vi "DEFINE_HMI_v2.0.vi"() -> ()   [LabVIEW 2020]
uses:
  <vilib>/userdefined/High Color/IMAQdx.ctl
  Keyence CL-3000/Public/clusters/CL3IF_MEASUREMENT_DATA.ctl
  Keyence CL-3000/Public/clusters/CL3IF_OUTMEASUREMENT_DATA.ctl
  Keyence CL-3000/Public/enums/CL3IF_VALUE_INFO.ctl
  Keyence CL-3000/Public/enums/CL3IF_JUDGE_RESULT.ctl
  Supporting Files/Sensor Station States.ctl
  Keyence CL-3000/Public/clusters/CL3IF_ETHERNET_SETTING.ctl
  4961857f-4cb1-4452-8877-0132d1278599.vi
  8fbe439c-06e5-460e-a560-e938ce784f44.vi
  460a15f0-0b3a-4794-87ef-3f3f720a4f09.vi
  13309ec4-5ddb-4caa-9ccb-149c6c5ba2b7.vi
  <vilib>/WebDAVClient/Advanced/Get File.vi
  <vilib>/Utility/inputDevices.llb/keyboardAcquire.vi
  <vilib>/Utility/inputDevices.llb/closeKeyboard.vi
  Keyence CL-3000/Keyence CL-3000.lvlib
  <vilib>/vision/driver/NI_Vision_Acquisition_Software.lvlib
  <vilib>/WebDAVClient/NI_WebDAV.lvlib
panel:
  out "Encoder Value":ext
  in  "Display Tab":enum32{"SENSOR FEEDBACK"}(tab)
  out "Chromatic Confocal":dbl(graph)
  out "Laser Displacement (cRIO)":dbl(graph)
  out "Captured Image":T1(plugin-control)
  out "Camera Feed":T1(plugin-control)
  in  "Motion Tab":enum32{"POSITION", "MEASUREMENT"}(tab)
  in  "Run Program":bool
  in  "Select Program":string(combo)="NONE"
  out "1st Key":T2(ring)
  in  "Bottom Button":bool
  in  "Top Button":bool
  in  "Next Button":bool
  in  "Previous Button":bool
  in  "Up Button":bool
  in  "Down Button":bool
  in  "Jog Axes":bool
  in  "Menu Ring":string(combo)
  in  "Move":bool
  in  "Axis 2 Distance":dbl format="%.2g"
  in  "Axis 1 Distance":dbl format="%.2g"
  in  "Axis 0 Distance":dbl format="%.2g"
  in  "Axis 0 Speed":dbl format="%.2g"
  in  "Axis 1 Speed":dbl format="%.2g"
  in  "Axis 2 Speed":dbl format="%.2g"
  in  "Axis 1 Acc":dbl format="%.2g"
  in  "Axis 0 Acc":dbl format="%.2g"
  in  "Axis 2 Acc":dbl format="%.2g"
  in  "Set Parameters 2":bool
  in  "Axis 2 Jogspeed":dbl format="%.2g"
  in  "Axis 1 Jogspeed":dbl format="%.2g"
  in  "Axis 0 Jogspeed":dbl format="%.2g"
  in  "Capture Image":bool
  in  "Sensor":i32(ring) items=["Chromatic", "Laser"]
  in  "Chromatic Data \nLogging":bool
  out "Logged Data Points":u32
  out "Index End":u32
  out "Index Start":u32
  out "Suffix":string
  in  "Measurement\nAxis":i32(ring) items=["X Axis", "Y Axis"]
  in  "Travel Speed\n(mm/s)":dbl format="%.2g"
  in  "Set Parameters":bool
  in  "Track Offset\n(mm)":dbl format="%.2g"
  in  "Ramp Distance\n(mm)":dbl min=0.0 format="%.2g"
  in  "Num Tracks":i32
  in  "Evaluation Length\n(mm)":dbl max=40.0 format="%.2g"
  in  "Test Name":string
  in  "Laser Data\nLogging":bool
  out "Travel Dist":dbl
  in  "Travel Acc\n(mm/s2)":dbl format="%.2g"
  in  "Start Measurement":bool
  in  "STOP":bool
  in  "Setup Tab":enum32{"SETUP", "MONITORING", "ERRORS"}(tab)
  in  "Home Axes":bool
  in  "Enable Camera":bool
  in  "Enable Laser":bool
  in  "Camera Input":T3
  in  "Enable Chromatic":bool
  in  "IP Address":u8[](array[numeric])=[192, 168, 1, 1]
  in  "Port":u32
  in  "Timeout":u32=5000
  in  "Comm Interface":enum8{"USB", "ETHERNET"}(ring)
  in  "Device ID":i32 min=0 max=2
  out "IsOpen":bool
  in  "Connection?":refnum<k7>(container)
  in  "Connect  to Controller":bool=TRUE
  in  "Set Parameters":bool
  in  "Controller Connection Type":string(combo)="2"
  out "Controller Type":string
  out "Product Name":string
  out "Version":string
  out "Serial Port":fxp<+,3,3>
  in  "Axis Enable":bool
  in  "Save Directory":path
  out "Z Error":bool
  out "Y Error":bool
  out "X Error":bool
  out "Axis 2 Velocity":dbl format="%.3g"
  out "Axis 2 End Pos":dbl format="%.3g"
  out "Axis 2 Position":dbl format="%.3g"
  out "Axis 0 Position":dbl format="%.3f"
  out "Axis 0 End Pos":dbl format="%.3g"
  out "Axis 0 Velocity":dbl format="%.3g"
  out "Axis 1 Position":dbl format="%.3g"
  out "Axis 1 Velocity":dbl format="%.3g"
  out "Axis 1 End Pos":dbl format="%.3g"
  out "A0 Remaining":dbl format="%.3g"
  out "A1 Remaining":dbl format="%.3g"
  out "A2 Remaining":dbl format="%.3g"
  out "Loop Time (us)":u32
  out "Measurement Data":T4(array[cluster])=[{"Out No"=1, "Value"=0, "valueInfo"=enum."VALID", "judgeResult"=0}, {"Out No"=2, "Value"=0, "valueInfo"=enum."VALID", "judgeResult"=0}, {"Out No"=3, "Value"=0, "valueInfo"=enum."VALID", "judgeResult"=0}, {"Out No"=4, "Value"=0, "valueInfo"=enum."VALID", "judgeResult"=0}, {"Out No"=5, "Value"=0, "valueInfo"=enum."VALID", "judgeResult"=0}, {"Out No"=6, "Value"=0, "valueInfo"=enum."VALID", "judgeResult"=0}, {"Out No"=7, "Value"=0, "valueInfo"=enum."VALID", "judgeResult"=0}, {"Out No"=8, "Value"=0, "valueInfo"=enum."VALID", "judgeResult"=0}] {"judgeResult" items=["HI"=1, "GO"=2, "LO"=4, "**"=5, "--"=0]}
  out "Total Time Elapsed (s)":i32
  out "XY Graph":cluster{"X":dbl, "Y":dbl}[](graph)
  out "Controller  Error":errorcluster
  out "Z Axis Error":errorcluster
  out "Y Axis Error":errorcluster
  out "X Axis Error":errorcluster
  out "Chromatic Sensor Error":errorcluster
  out "Laser Sensor Error":errorcluster
  # "SET PARAMETERS"
  # "DIRECT MOTION"
  # "SPEED \n(mm/s)"
  # "ACC / DEC\n(mm/s2)"
  # "JOGSPEED \n(mm/s)"
  # "X AXIS"
  # "X AXIS"
  # "(mm)"
  # "Y AXIS"
  # "Y AXIS"
  # "(mm)"
  # "Z AXIS"
  # "Z AXIS"
  # "(mm)"
  # "AXIS JOGGING"
  # "XY AXES"
  # "Z AXIS"
  # "KEYBOARD"
  # "CONTROLLER PROGRAMS"
  # "Suffix will be auto-genereated for each measurement e.g. Test Name_01, Test Name_02, etc."
  # "MEASUREMENT PARAMETERS"
  # "CHROMATIC CONFOCAL"
  # "LASER DISPLACEMENT"
  # "CAMERA"
  # "CONTROLLER SETTINGS"
  # "CHROMATIC CONFOCAL SETTINGS"
  # "LASER DISPLACEMENT SETTINGS"
  # "CAMERA SETTINGS"
  # "AXIS FEEDBACK"
  # "Current Position \n(mm)"
  # "End Position \n(mm)"
  # "Travel Remaining \n(mm)"
  # "Velocity \n(mm/s2)"
  # "X AXIS"
  # "Y AXIS"
  # "Z AXIS"
  # "CONTROLLER"
  # "CHROMATIC CONFOCAL"
  # "CONTROLLER"
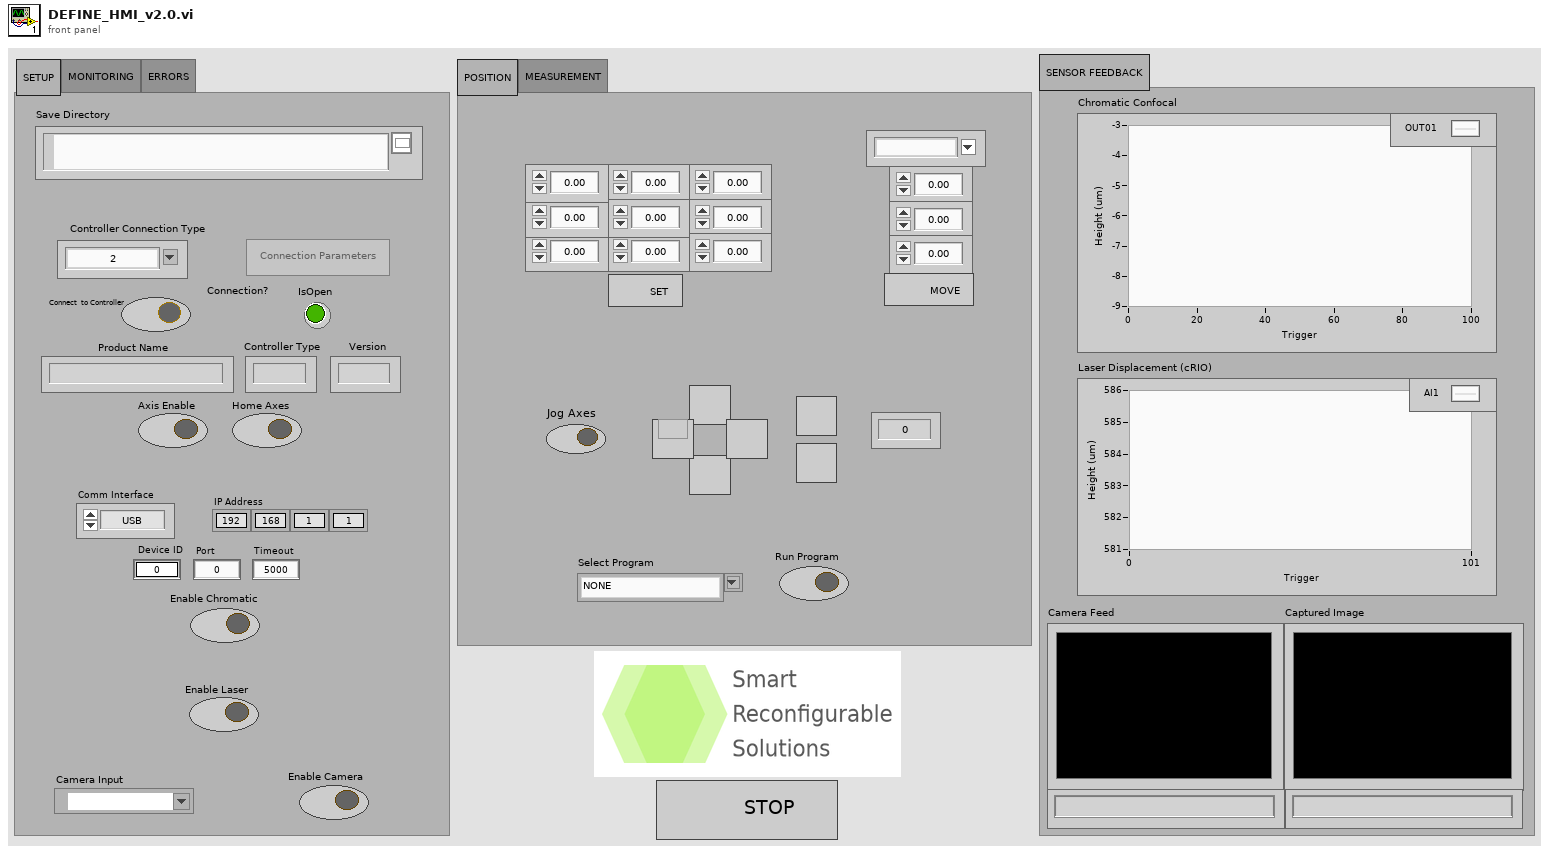
[diagram p1: front panel]
types:
  T1 = typedef "IMAQ Image.ctl" = refnum<image>
  T2 = enum16{"0", "1", "2", "3", "4", "5", "6", "7", "8", "9", "A", "B", "C", "D", "E", "F", "G", "H", "I", "J", "K", "L", "M", "N", "O", "P", "Q", "R", "S", "T", "U", "V", "W", "X", "Y", "Z", "F1", "F2", "F3", "F4", "F5", "F6", "F7", "F8", "F9", "F10", "F11", "F12", "F13", "F14", "F15", "ADD", "BACK", "BACKSLASH", "CAPITAL", "COMMA", "DECIMAL", "DELETE", "DIVIDE", "DOWN", "END", "EQUALS", "ESCAPE", "GRAVE (`)", "HOME", "INSERT", "LBRACKET", "LCONTROL", "LEFT", "L ALT", "LSHIFT", "LWIN", "MINUS", "MULTIPLY", "NEXT", "NUMLOCK", "NUMPAD_0", "NUMPAD_1", "NUMPAD_2", "NUMPAD_3", "NUMPAD_4", "NUMPAD_5", "NUMPAD_6", "NUMPAD_7", "NUMPAD_8", "NUMPAD_9", "PAUSE", "PERIOD", "PRIOR (PG UP)", "RBRACKET", "RCONTROL", "RETURN", "RIGHT", "R ALT", "RSHIFT", "RWIN", "SCROLL", "SEMICOLON", "SLASH", "SPACE", "SUBTRACT", "TAB", "UP", "ENTER (num pad)", "' (quote)"}
  T3 = typedef "IMAQdx.ctl" = refnum<k21>
  T4 = cluster{"Out No":i32, "Value":i32, "valueInfo":enum8{"VALID", "JUDGMENTSTANDBY", "INVALID", "OVERDISPRANGE_P", "OVERDISPRANGE_N"}, "judgeResult":u16}[]
  T5 = typedef "Sensor Station States.ctl" = enum16{"Initialise", "Acquire", "Visualise", "Log", "Save", "Check Time", "Idle", "Close"}
  T6 = enum16{"open", "replace", "create", "open or create", "replace or create", "replace or create with confirmation"}
  T7 = typedef "Keyence CL-3000.lvlib/CL3IF_ETHERNET_SETTING.ctl" = cluster{"IP Address":cluster{"IP1":u8, "IP2":u8, "IP3":u8, "IP4":u8}, "portNo":u32}
  T8 = typedef "Keyence CL-3000.lvlib/CL3IF_MEASUREMENT_DATA.ctl" = cluster{"addInfo":cluster{"triggerCount":u32, "pulseCount":i32}, "outMeasurementData":T9[]}
  T9 = typedef "Keyence CL-3000.lvlib/CL3IF_OUTMEASUREMENT_DATA.ctl" = cluster{"measurementValue":i32, "valueInfo":T10, "judgeResult":T11}
  T10 = typedef "Keyence CL-3000.lvlib/CL3IF_VALUE_INFO.ctl" = enum8{"VALID", "JUDGMENTSTANDBY", "INVALID", "OVERDISPRANGE_P", "OVERDISPRANGE_N"}
  T11 = typedef "Keyence CL-3000.lvlib/CL3IF_JUDGE_RESULT.ctl" = u8
  T12 = cluster{"IP Address":u8, "IP Address":u8, "IP Address":u8, "IP Address":u8}
  T13 = cluster{i32, "measurementValue":i32, "valueInfo":T10, "judgeResult":T11}
  T14 = typedef "NI_WebDAV.lvlib/SessionHandle.ctl" = refnum<k1>
  T15 = enum16{"0", "1", "2", "3", "4", "5", "6", "7", "8", "9", "A", "B", "C", "D", "E", "F", "G", "H", "I", "J", "K", "L", "M", "N", "O", "P", "Q", "R", "S", "T", "U", "V", "W", "X", "Y", "Z", "F1", "F2", "F3", "F4", "F5", "F6", "F7", "F8", "F9", "F10", "F11", "F12", "F13", "F14", "F15", "ADD", "BACK", "BACKSLASH", "CAPITAL", "COMMA", "DECIMAL", "DELETE", "DIVIDE", "DOWN", "END", "EQUALS", "ESCAPE", "GRAVE (`)", "HOME", "INSERT", "LBRACKET", "LCONTROL", "LEFT", "L ALT", "LSHIFT", "LWIN", "MINUS", "MULTIPLY", "NEXT", "NUMLOCK", "NUMPAD_0", "NUMPAD_1", "NUMPAD_2", "NUMPAD_3", "NUMPAD_4", "NUMPAD_5", "NUMPAD_6", "NUMPAD_7", "NUMPAD_8", "NUMPAD_9", "PAUSE", "PERIOD", "PRIOR (PG UP)", "RBRACKET", "RCONTROL", "RETURN", "RIGHT", "R ALT", "RSHIFT", "RWIN", "SCROLL", "SEMICOLON", "SLASH", "SPACE", "SUBTRACT", "TAB", "UP", "ENTER (num pad)", "' (quote)"}[]
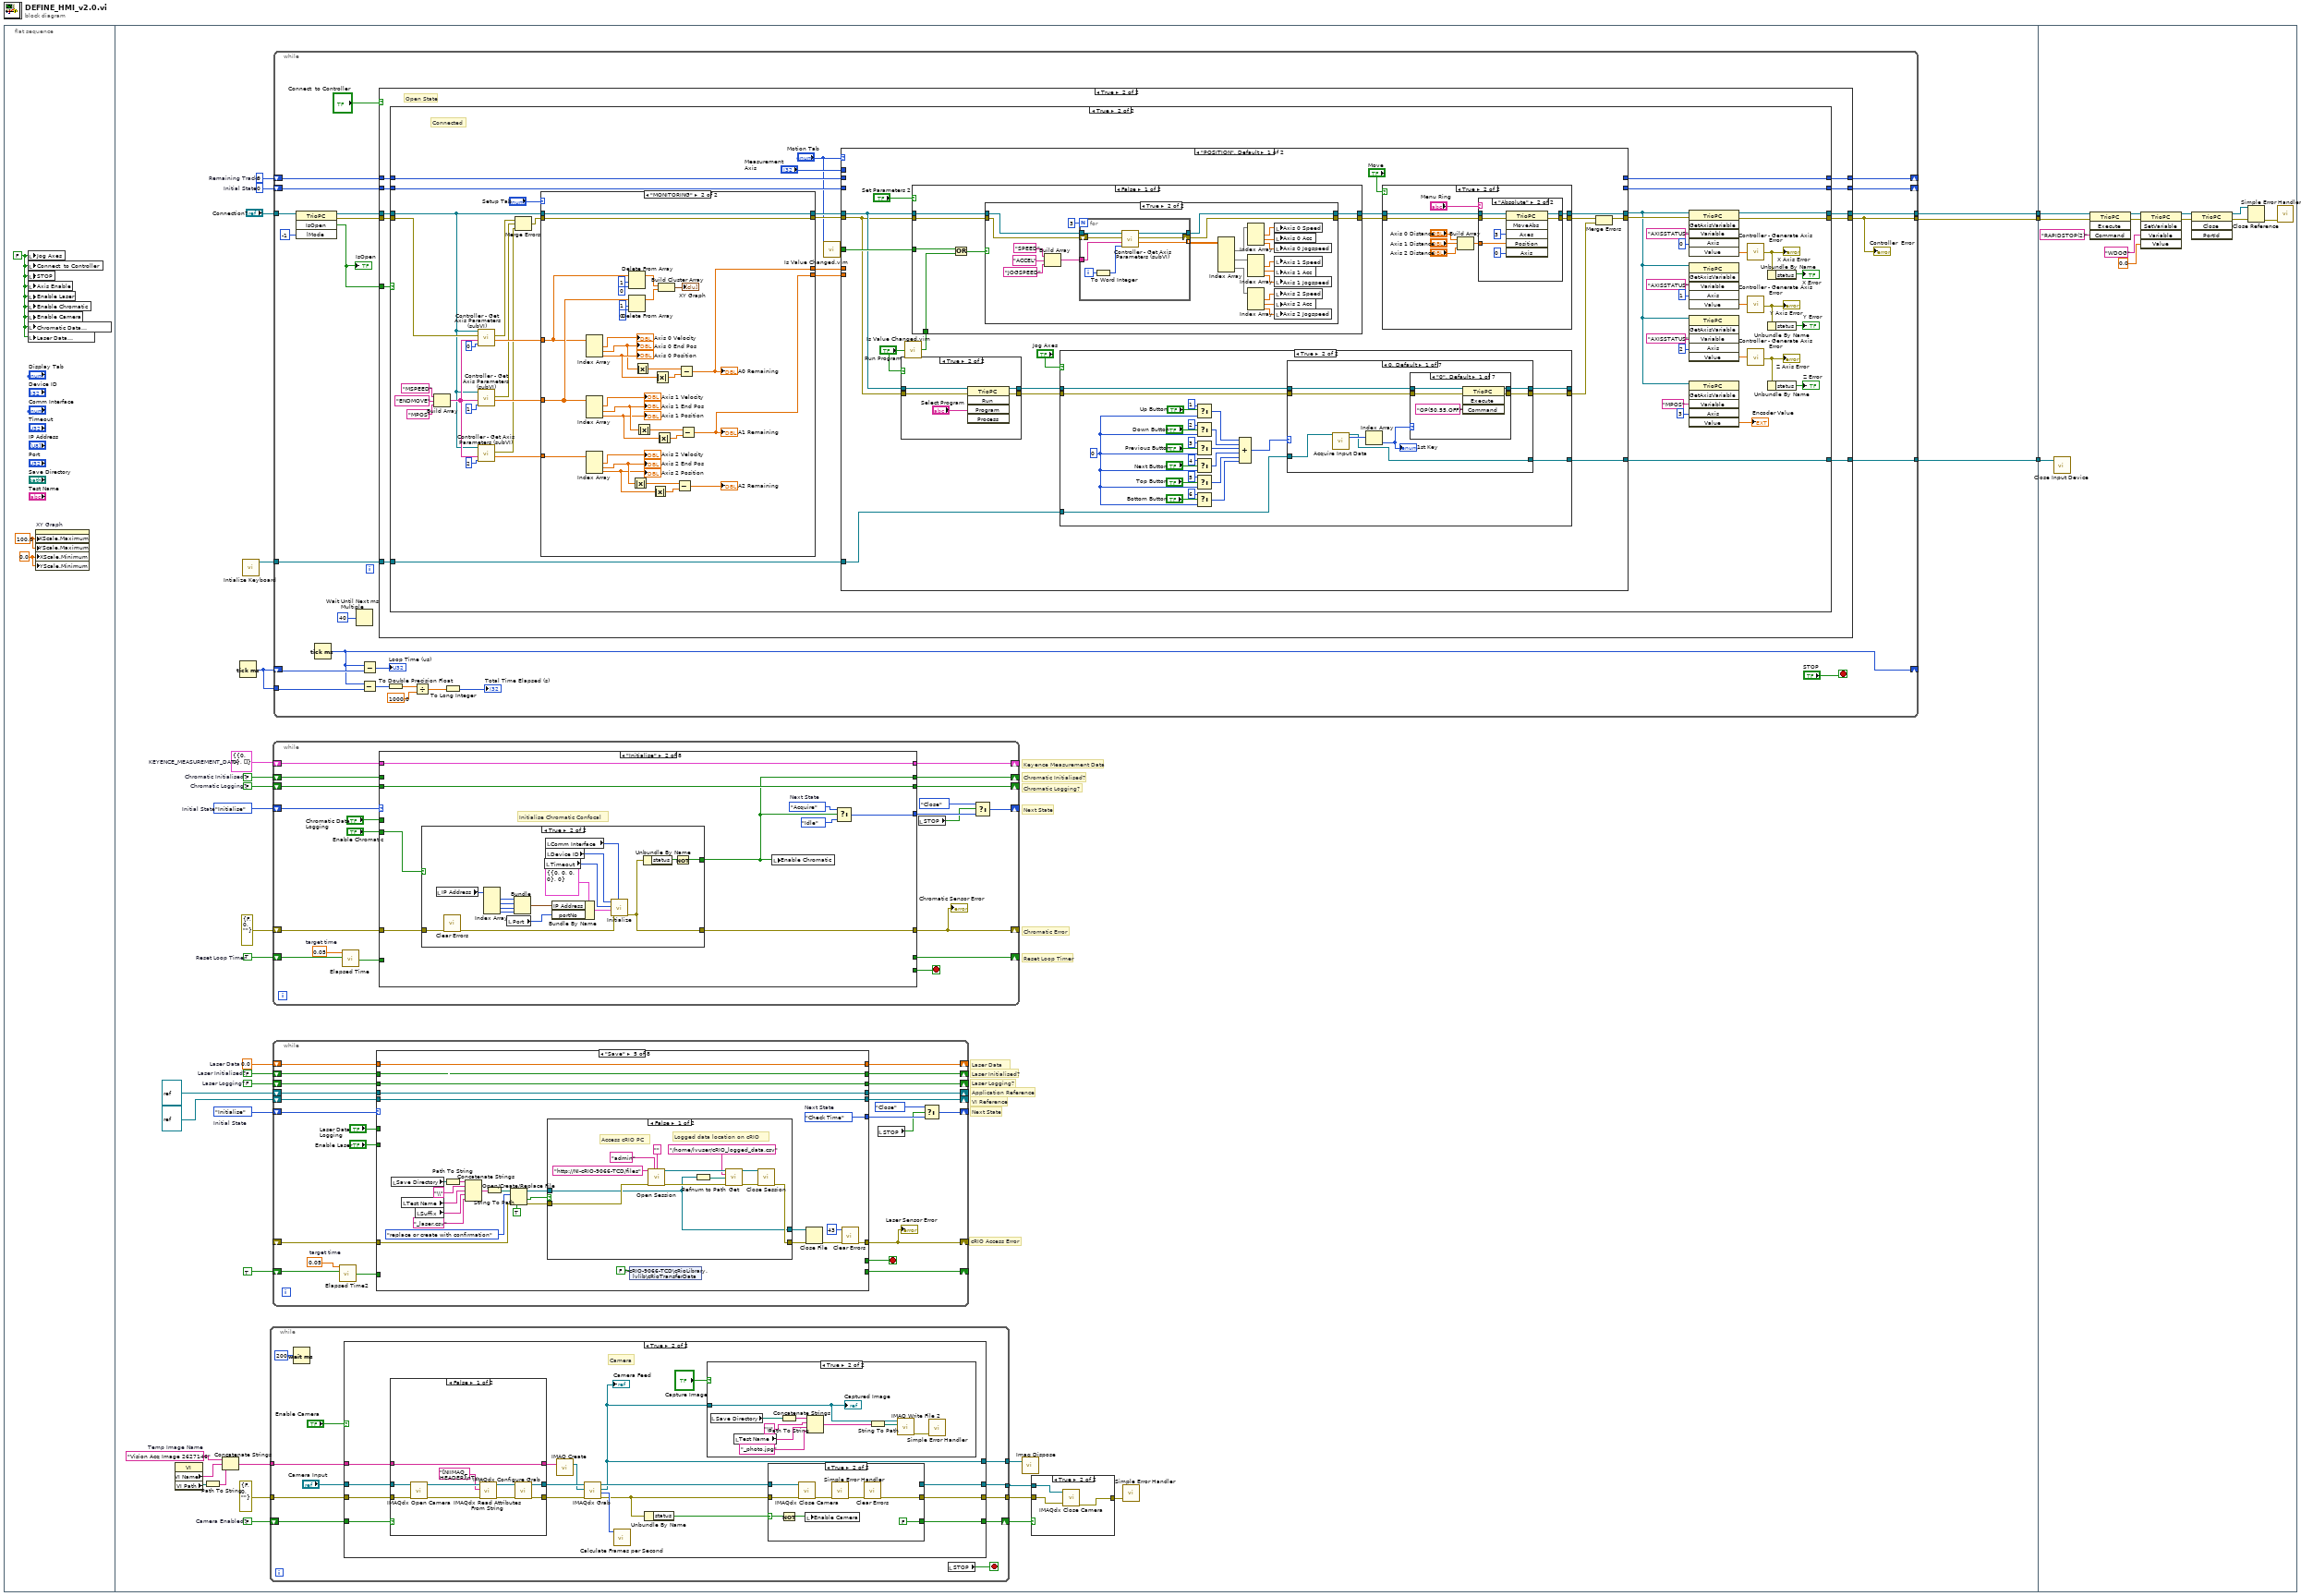
[diagram p0: block diagram]
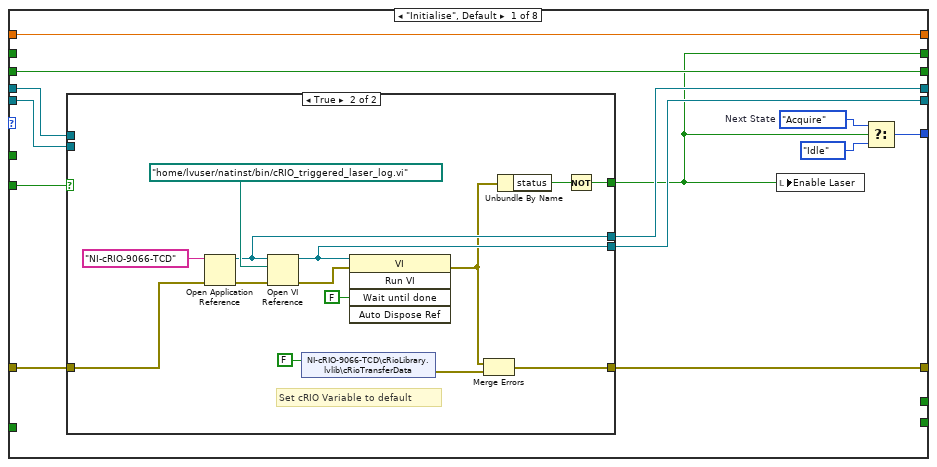
[diagram p2: hidden frame]
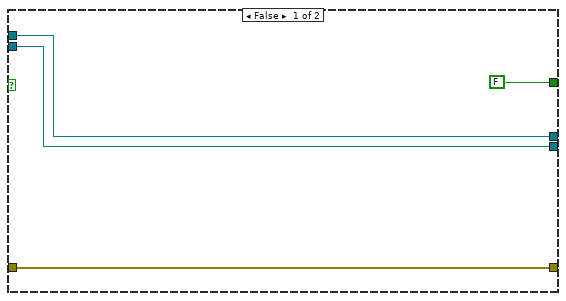
[diagram p3: hidden frame]
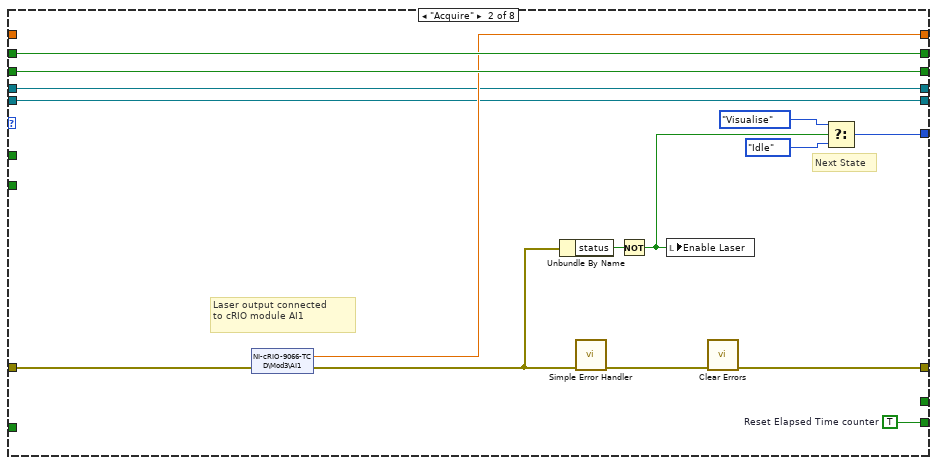
[diagram p4: hidden frame]
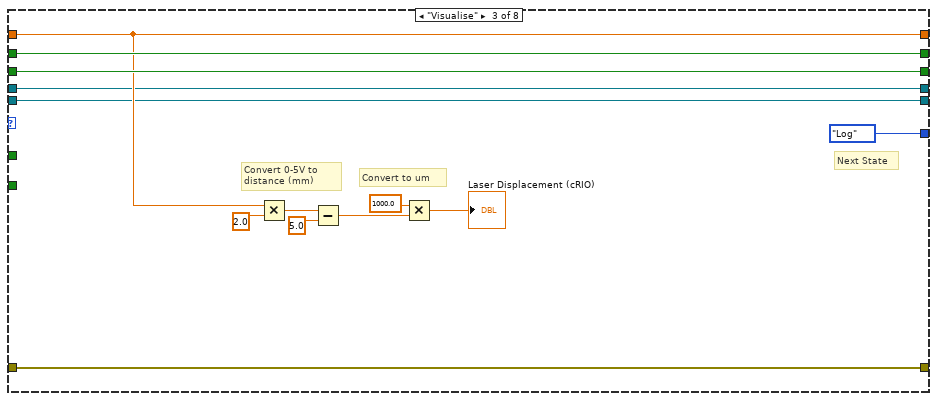
[diagram p5: hidden frame]
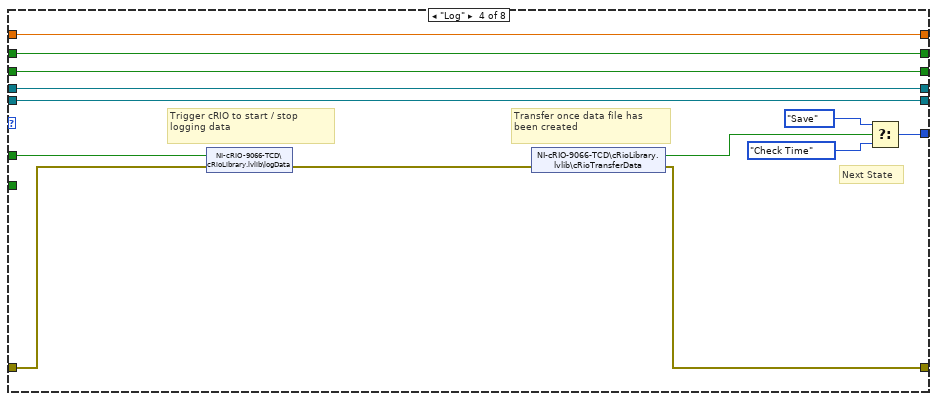
[diagram p6: hidden frame]
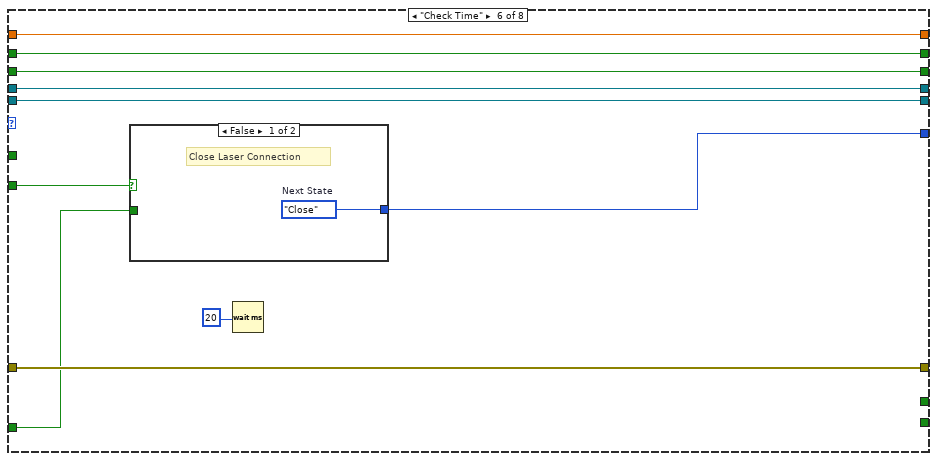
[diagram p8: hidden frame]
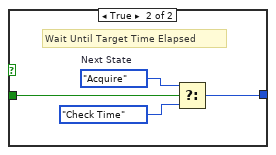
[diagram p9: hidden frame]
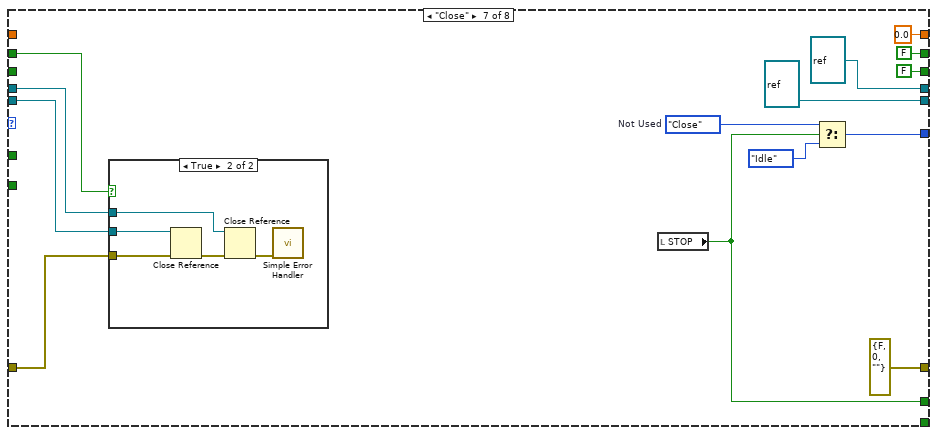
[diagram p10: hidden frame]
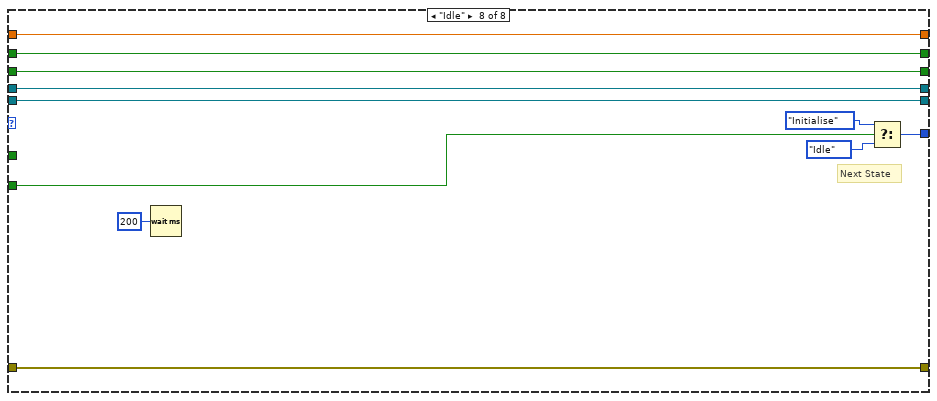
[diagram p12: hidden frame]
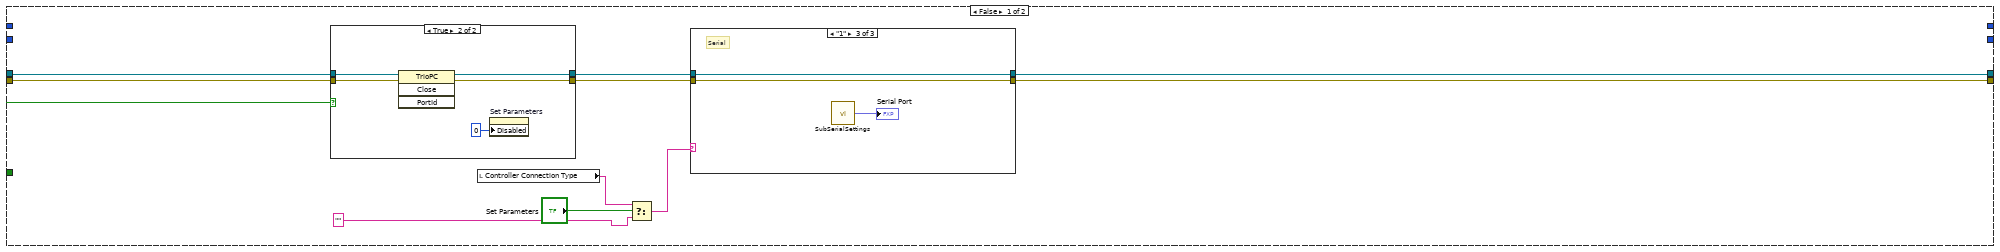
[diagram p13: hidden frame]
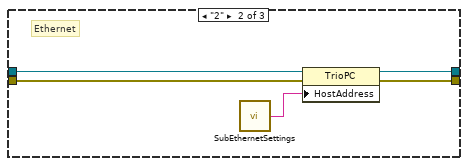
[diagram p16: hidden frame]
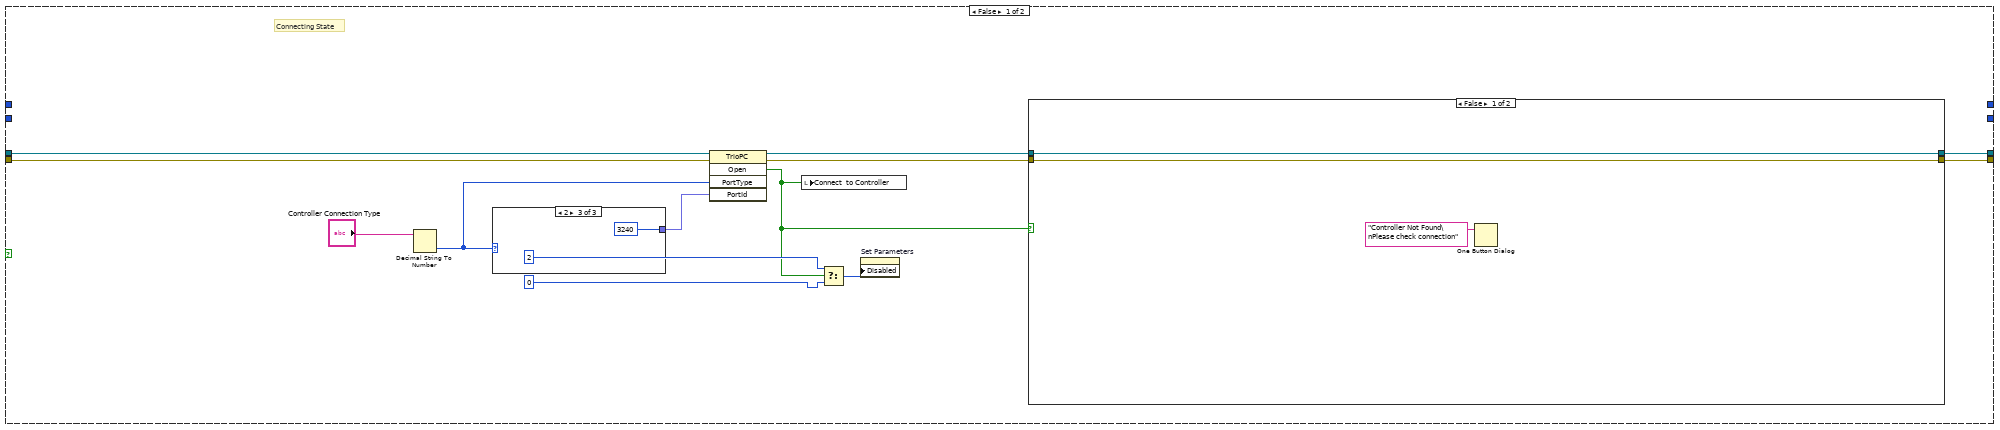
[diagram p17: hidden frame]
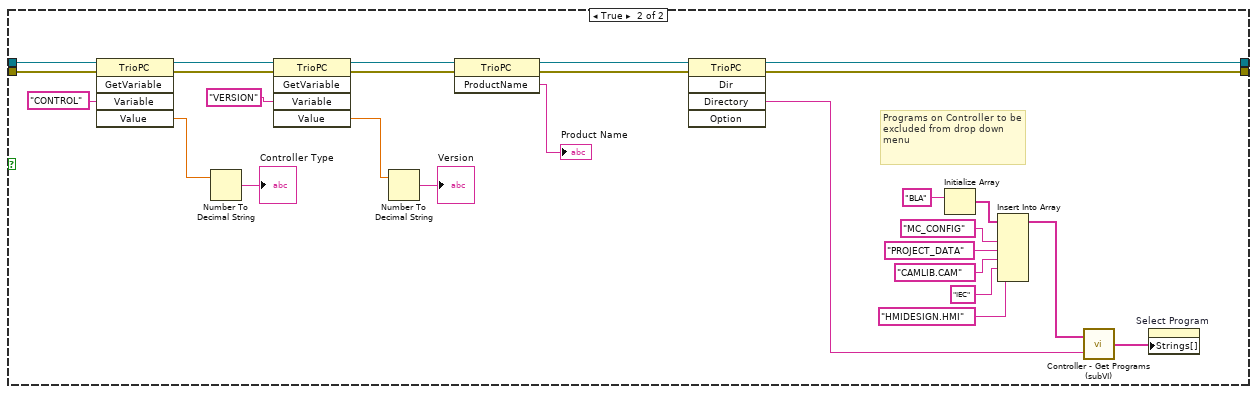
[diagram p18: hidden frame]
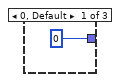
[diagram p19: hidden frame]
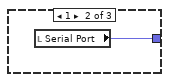
[diagram p20: hidden frame]
diagram:
  n1 = flat-sequence {
    tunnel: [w38] -> w3
    tunnel: [w37] -> w2
    tunnel: [w34] -> w1
    tunnel: w3 -> [w1152]
    tunnel: w2 -> [w1153]
    tunnel: w1 -> [w1154]
    frame #0 {
      w6 = 0.0 ("X Scale.Range:Minimum")
      w5 = 100.0 ("X Scale.Range:Maximum")
      w4 = FALSE ("Jog Axes")
      n2 = local write "Jog Axes"(w4) -> ()
      n3 = local write "Connect  to Controller"(w4) -> ()
      n4 = local write "STOP"(w4) -> ()
      n5 = local write "Axis Enable"(w4) -> ()
      n6 = local write "Enable Laser"(w4) -> ()
      n7 = local write "Enable Chromatic"(w4) -> ()
      n8 = local write "Enable Camera"(w4) -> ()
      n9 = local write "Chromatic Data \nLogging"(w4) -> ()
      n10 = local write "Laser Data\nLogging"(w4) -> ()
      n11 = property on="XY Graph" class="XYGraph (strict)"("XScale.Maximum"=w5, "YScale.Maximum"=w5, "XScale.Minimum"=w6, "YScale.Minimum"=w6) -> ()  [unwired: 2 in, 2 out]
    }
    frame #1 {
      w9 = 0.0  # Laser Data
      w10 = FALSE  # Laser Initialised?
      w13 = FALSE  # Laser Logging?
      w11 = Sensor_Station_States."Initialise"  # Initial State
      w14 = 0  # Remaining Tracks
      w15 = 0  # Initial State
      w18 = "Vision Acq Image 2627146"  # Temp Image Name
      w17 = FALSE  # Camera Enabled?
      w28 = FALSE  # Chromatic Initialised?
      w30 = FALSE  # Chromatic Logging?
      w31 = TRUE  # Reset Loop Timer
      w32 = T8 {"addInfo"={"triggerCount"=0, "pulseCount"=0}, "outMeasurementData"=[]}  # KEYENCE_MEASUREMENT_DATA
      w33 = Sensor_Station_States."Initialise"  # Initial State
      # "VI Reference"
      # "Application Reference"
      # "cRIO Access Error"
      # "Next State"
      # "Laser Logging?"
      # "Laser Initialised?"
      # "Laser Data"
      # "Reset Loop Timer"
      # "Chromatic Error"
      # "Next State"
      # "Keyence Measurement Data"
      # "Chromatic Logging?"
      # "Chromatic Initialised?"
      n12 = property class="VI"() -> ("VI Name"=w21:string, "VI Path"=w22:path)  [unwired: 2 in, 2 out]
      n13 = Path To String(path=w22) -> (string=w20:string)
      n14 = Concatenate Strings(w18, w21, w20) -> (w23:string)
      n15 = Tick Count (ms)() -> (millisecond timer value=w36:u32)
      n16 = call <vilib>:"Intialize Keyboard.vi"() -> ("device ID"=w35:refnum<k1>)  [unwired: 1 in, 10 out]
      n17 = while {
        tunnel: [w901] -> w19
        tunnel: [w900] -> w25
        shift-right: [w892] -> w27
        shift-left: w17 -> [w896]
        tunnel: errorcluster {"status"=FALSE, "code"=0, "source"=""} ("error in") -> [w894]
        tunnel: w23 -> [w895]
        tunnel: [w891] -> w24
        stop <- w897 stop-if-true
        n18 = Wait (ms)(milliseconds to wait=u32 200) -> ()  [unwired: 1 out]
        n19 = case shown="True" "Enable Camera" {
          tunnel: [w903 w920] -> w900
          tunnel: [_ w914] -> w901
          tunnel: w896 -> [w902 w913]
          tunnel: w895 -> [_ w909]
          tunnel: w894 -> [w903 w912]
          tunnel: "Camera Input" -> [w904 w908]
          tunnel: [w902 w906] -> w892
          tunnel: [w904 w905] -> w891
          frame False {
          }
          frame True {
            # "Camera"
            n20 = case shown="False" w913 {
              tunnel: [w931 w933] -> w916
              tunnel: [w930 w932] -> w915
              tunnel: w912 -> [w925 w932]
              tunnel: [w924 w934] -> w910
              tunnel: w909 -> [w924 w934]
              tunnel: w908 -> [w923 w933]
              frame False {
                n21 = call <vilib>:"IMAQdx Open Camera.vi"("error in"=w925, "Session In"=w923) -> ("error out"=w928:errorcluster, "Session Out"=w929:T3)  [unwired: 1 in, 7 out]
                n22 = call <vilib>:"IMAQdx Read Attributes From String.vi"("error in"=w928, "Attributes String In"="[NIIMAQ_HEADER]\nType = 2\nVersion = 8\n\n[CAMERA_DATA]\nAcquisitionAttributes::Bayer::Algorithm = \"Bilinear\"\nAcquisitionAttributes::Bayer::GainB = \"1\"\nAcquisitionAttributes::Bayer::GainG = \"1\"\nAcquisitionAttributes::Bayer::GainR = \"1\"\nAcquisitionAttributes::Bayer::Pattern = \"Use hardware value\"\nAcquisitionAttributes::BitsPerPixel = \"Use hardware value\"\nAcquisitionAttributes::HardwareMaximumQueuedBufferCount = \"1000\"\nAcquisitionAttributes::HardwareRequeueBufferListThreshold = \"50\"\nAcquisitionAttributes::IgnoreFirstFrame = \"false\"\nAcquisitionAttributes::ImageDecoderCopyMode = \"Auto\"\nAcquisitionAttributes::OutputImageType = \"Auto\"\nAcquisitionAttributes::OverwriteMode = \"Get Newest\"\nAcquisitionAttributes::PixelSignedness = \"Use hardware value\"\nAcquisitionAttributes::ReceiveTimestampMode = \"None\"\nAcquisitionAttributes::ShiftPixelBits = \"false\"\nAcquisitionAttributes::SwapPixelBytes = \"false\"\nAcquisitionAttributes::Timeout = \"5000\"\nAcquisitionAttributes::VerticalMirror = \"false\"\nAcquisitionAttributes::VideoMode = \"640x480 YUY2 30.00fps\"\nCameraAttributes::BacklightCompensation::Mode = \"Manual\"\nCameraAttributes::BacklightCompensation::Value = \"true\"\nCameraAttributes::Brightness::Mode = \"Manual\"\nCameraAttributes::Brightness::Value = \"0\"\nCameraAttributes::Contrast::Mode = \"Manual\"\nCameraAttributes::Contrast::Value = \"0.179999999999999993\"\nCameraAttributes::Exposure::Mode = \"Auto\"\nCameraAttributes::Gain::Mode = \"Manual\"\nCameraAttributes::Gain::Value = \"1\"\nCameraAttributes::Gamma::Mode = \"Manual\"\nCameraAttributes::Gamma::Value = \"1.5\"\nCameraAttributes::Hue::Mode = \"Manual\"\nCameraAttributes::Hue::Value = \"0\"\nCameraAttributes::Saturation::Mode = \"Manual\"\nCameraAttributes::Saturation::Value = \"8\"\nCameraAttributes::Sharpness::Mode = \"Manual\"\nCameraAttributes::Sharpness::Value = \"3\"\nCameraAttributes::WhiteBalance::Mode = \"Auto\"\n" ("Attributes"), "Session In"=w929) -> ("error out"=w926:errorcluster, "Session Out"=w927:T3)  [unwired: 7 out]
                n23 = call <vilib>:"IMAQdx Configure Grab.vi"("error in"=w926, "Session In"=w927) -> ("error out"=w930:errorcluster, "Session Out"=w931:T3)  [unwired: 1 in, 7 out]
              }
              frame True {
                # "Camera Initialised"
              }
            }
            n24 = call "IMAQ Create"("Image Name"=w910) -> ("New Image"=w911:T1)  [unwired: 3 in, 2 out]
            n25 = call <vilib>:"IMAQdx Grab.vi"("error in"=w915, "Image In"=w911, "Session In"=w916) -> ("error out"=w917:errorcluster, "Buffer Number Out"=w918:u32, "Image Out"=w914:T1, "Session Out"=w919:T3)  [unwired: 1 in, 4 out]
            "Camera Feed" <- w914
            n26 = call <vilib>:"Calculate Frames per Second.vi"("Buffer Number"=w918) -> ()  [unwired: 2 in, 9 out]
            n27 = Unbundle By Name(w917) -> ("status"=w907:bool)
            n28 = case shown="True" "Capture Image" {
              tunnel: w914 -> [_ w954]
              frame False {
              }
              frame True {
                n29 = local read "Save Directory"() -> (w950:path)
                n30 = local read "Test Name"() -> (w952:string)
                n31 = Path To String(path=w950) -> (string=w951:string)
                n32 = Concatenate Strings(w951, "\\" ("string"), w952, "_photo.jpg" ("string")) -> (w949:string)
                n33 = String To Path(string=w949) -> (path=w946:path)
                n34 = call-poly "IMAQ Write File 2"("File Path"=w946, "Image"=w954) -> ("error out"=w953:errorcluster)  [unwired: 8 in, 1 out]
                n35 = call <vilib>:"Simple Error Handler.vi"("error in (no error)"=w953) -> ()  [unwired: 4 in, 5 out]
                "Captured Image" <- w954
              }
            }
            n36 = case "Case Structure_template1" shown="True" w907 {
              selector: w907 -> [_ w940]
              tunnel: [w937 w941] -> w920
              tunnel: w917 -> [w937 w945]
              tunnel: w919 -> [w935 w943]
              tunnel: [TRUE FALSE] -> w906
              tunnel: [w935 _] -> w905
              frame False {
              }
              frame True {
                n37 = Not(x=w940) -> (.not. x?=w939:bool)
                n38 = call <vilib>:"IMAQdx Close Camera.vi"("error in"=w945, "Session In"=w943) -> ("error out"=w944:errorcluster)  [unwired: 9 out]
                n39 = local write "Enable Camera"(w939) -> ()
                n40 = call <vilib>:"Simple Error Handler.vi"("error in (no error)"=w944) -> ("error out"=w942:errorcluster)  [unwired: 4 in, 4 out]
                n41 = call <vilib>:"Clear Errors.vi"("error in (no error)"=w942) -> ("error out"=w941:errorcluster)  [unwired: 5 in, 1 out]
              }
            }
          }
        }
        n42 = local read "STOP"() -> (w897:bool)
      }
      n43 = while {
        shift-right: [w960] -> _
        shift-left: w33 -> [w974]
        shift-right: [w972] -> _
        shift-left: w32 -> [w973]
        shift-right: [w968] -> _
        shift-left: w31 -> [w970]
        shift-right: [w966] -> _
        shift-left: w30 -> [w967]
        shift-right: [w955] -> _
        shift-left: errorcluster {"status"=FALSE, "code"=0, "source"=""} ("error constant") -> [w965]
        shift-right: [w964] -> _
        shift-left: w28 -> [w963]
        stop <- w959 stop-if-true
        w971 = 0.05  # target time
        n44 = call "Elapsed Time"("Time Target (s)"=w971, "Reset"=w970) -> ("Time has Elapsed"=w969:bool)  [unwired: 10 in, 7 out]
        n45 = case shown="\"Initialise\"" w974 {
          tunnel: w973 -> [w982 w992 _ w1028 w1047 w1095 w1120 _]
          tunnel: w965 -> [w976 w988 w1017 w1031 w1050 w1081 w1123 w1141]
          tunnel: [w982 w992 w1013 w1028 w1047 w1095 w1120 T8 {"addInfo"={"triggerCount"=0, "pulseCount"=0}, "outMeasurementData"=[]} ("KEYENCE_MEASUREMENT_DATA")] -> w972
          tunnel: [w979 w990 w1016 Sensor_Station_States."Log" ("Next State") w1043 w1086 w1121 w1135] -> w962
          tunnel: w969 -> [_ _ _ _ _ _ w1122 _]
          tunnel: [_ _ w1019 _ _ _ _ _] -> w968
          tunnel: w967 -> [w975 w989 w1018 w1030 w1051 w1084 w1125 _]
          tunnel: [w975 w989 w1018 w1030 w1049 w1084 w1125 FALSE ("Chromatic Logging?")] -> w966
          tunnel: [w976 w984 w1014 w1031 w1040 w1082 w1123 errorcluster {"status"=FALSE, "code"=0, "source"=""} ("error constant")] -> w955
          tunnel: [w983 w985 w1012 w1032 w1048 w1085 w1124 FALSE] -> w964
          tunnel: w963 -> [w983 _ w1012 w1032 w1048 w1085 w1124 w1134]
          tunnel: [_ _ _ _ _ _ _ w1132] -> w959
          tunnel: "Enable Chromatic" -> [w978 w986 _ _ _ _ w1119 _]
          tunnel: "Chromatic Data \nLogging" -> [_ _ _ _ w1042 _ _ _]
          frame "Idle", Default {
            w981 = Sensor_Station_States."Initialise"  # Next State
            n46 = Wait (ms)(milliseconds to wait=u32 200) -> ()  [unwired: 1 out]
            n47 = Select(t=w981, s=w978, f=Sensor_Station_States."Idle" ("Next State")) -> (s? t:f=w979:T5)
          }
          frame "Initialise" {
            w991 = Sensor_Station_States."Acquire"  # Next State
            # "Initialise Chromatic Confocal"
            n48 = case shown="True" w986 {
              tunnel: [w993 w998] -> w984
              tunnel: [FALSE w997] -> w985
              tunnel: w988 -> [w993 w999]
              frame False {
              }
              frame True {
                n49 = local read "IP Address"() -> (w1001:u8[])
                n50 = call <vilib>:"Clear Errors.vi"("error in (no error)"=w999) -> ("error out"=w995:errorcluster)  [unwired: 5 in, 1 out]
                n51 = Index Array(array=w1001) -> (element #1=w1006:u8, element #2=w1007:u8, element #3=w1008:u8, element #4=w1009:u8)  [unwired: 4 in]
                n52 = local read "Port"() -> (w1000:u32)
                n53 = Bundle("IP Address"=w1006, "IP Address"=w1007, "IP Address"=w1008, "IP Address"=w1009) -> (w1010:T12)  [unwired: 1 in]
                n54 = local read "Timeout"() -> (w1002:u32)
                n55 = local read "Comm Interface"() -> (w1003:enum8{"USB", "ETHERNET"})
                n56 = local read "Device ID"() -> (w1004:i32)
                n57 = Bundle By Name(cluster=T7 {"IP Address"={"IP1"=0, "IP2"=0, "IP3"=0, "IP4"=0}, "portNo"=0} ("ethernetSetting"), "IP Address"=w1010, "portNo"=w1000) -> (w1011:T7)
                n58 = call "Initialize.vi"("Comm Interface"=w1003, "error in (no error)"=w995, "ethernetSetting"=w1011, "timeout"=w1002, "deviceId"=w1004) -> ("error out"=w998:errorcluster)  [unwired: 6 in]
                n59 = Unbundle By Name(w998) -> ("status"=w996:bool)
                n60 = Not(x=w996) -> (.not. x?=w997:bool)
              }
            }
            n61 = local write "Enable Chromatic"(w985) -> ()
            n62 = Select(t=w991, s=w985, f=Sensor_Station_States."Idle" ("Next State")) -> (s? t:f=w990:T5)
          }
          frame "Acquire" {
            w1016 = Sensor_Station_States."Visualise"  # Next State
            w1019 = TRUE  # Reset Elapsed Time counter
            n63 = local read "Device ID"() -> (w1015:i32)
            n64 = call "CL3IF_GetMeasurementData.vi"("error in"=w1017, "deviceId"=w1015) -> ("error out"=w1014:errorcluster, "MEASUREMENT_DATA"=w1013:T8)  [unwired: 8 in]
          }
          frame "Visualise" {
            n65 = Unbundle By Name(w1028) -> ("outMeasurementData"=w1026:T9[])
            n66 = Index Array(array=w1026, index=0) -> (element=w1025:T9)
            n67 = for {
              tunnel: w1026 -> [w1039] mode=indexing
              tunnel: [w1038] -> w1027 mode=indexing
              i -> [w1037]
              n68 = Unbundle By Name(w1039) -> ("measurementValue"=w1033:i32, "valueInfo"=w1035:T10, "judgeResult"=w1034:T11)
              n69 = Increment(x=w1037) -> (x+1=w1036:i32)
              n70 = Bundle(w1036, "measurementValue"=w1033, "valueInfo"=w1035, "judgeResult"=w1034) -> (w1038:T13)  [unwired: 1 in]
            }
            "Measurement Data" <- w1027
            n71 = Unbundle By Name(w1025) -> ("measurementValue"=w1024:i32)
            n72 = To Double Precision Float(number=w1024) -> (double precision float=w1020:dbl)
            n73 = Divide(x=w1020, y=1000.0) -> (x/y=→"Chromatic Confocal":dbl)
          }
          frame "Log" {
            w1045 = Sensor_Station_States."Save"  # Next State
            n74 = local read "Device ID"() -> (w1041:i32)
            n75 = case shown="False" w1042 {
              tunnel: w1051 -> [w1056 w1070]
              tunnel: w1050 -> [w1057 w1069]
              tunnel: [w1055 w1068] -> w1040
              tunnel: [FALSE TRUE] -> w1049
              tunnel: [w1053 FALSE ("conSaveData")] -> w1046
              tunnel: w1041 -> [w1052 w1065]
              frame False {
                n76 = case shown="True" w1056 {
                  tunnel: w1057 -> [w1059 w1063]
                  tunnel: [w1059 w1061] -> w1055
                  tunnel: [FALSE ("conSaveData") TRUE ("conSaveData")] -> w1053
                  tunnel: w1052 -> [_ w1060]
                  frame False {
                    # "Not Logging\nDo nothing"
                  }
                  frame True {
                    # "Move to Save State"
                    # "Stop Logging & Record Data Index"
                    n77 = call "CL3IF_GetTrendIndex.vi"("error in"=w1063, "deviceId"=w1060) -> ("error out"=w1061:errorcluster, "index"=→"Index End":u32)  [unwired: 8 in]
                  }
                }
              }
              frame True {
                n78 = case shown="False" w1070 {
                  tunnel: w1069 -> [w1073 w1075]
                  tunnel: [w1072 w1075] -> w1068
                  tunnel: w1065 -> [w1071 _]
                  frame False {
                    # "Start Logging"
                    n79 = call "CL3IF_GetTrendIndex.vi"("error in"=w1073, "deviceId"=w1071) -> ("error out"=w1072:errorcluster, "index"=→"Index Start":u32)  [unwired: 8 in]
                  }
                  frame True {
                    # "Currently Logging\nDo nothing"
                  }
                }
              }
            }
            n80 = Select(t=w1045, s=w1046, f=Sensor_Station_States."Check Time" ("Next State")) -> (s? t:f=w1043:T5)
          }
          frame "Save" {
            w1086 = Sensor_Station_States."Check Time"  # Next State
            n81 = local read "Save Directory"() -> (w1092:path)
            n82 = local read "Index Start"() -> (w1094:u32)
            n83 = local read "Index End"() -> (w1093:u32)
            n84 = local read "Test Name"() -> (w1089:string)
            n85 = local read "Suffix"() -> (w1076:string)
            n86 = local read "Device ID"() -> (w1083:i32)
            n87 = Path To String(path=w1092) -> (string=w1091:string)
            n88 = Concatenate Strings(w1091, "\\" ("string"), w1089, w1076, "_confocal.csv" ("string")) -> (w1088:string)
            n89 = Subtract(x=w1093, y=w1094) -> (x-y=w1102:u32)
            "Logged Data Points" <- w1102
            n90 = String To Path(string=w1088) -> (path=w1087:path)
            n91 = call "CL3IF_GetTrendData.vi"("requestDataCount"=w1102, "index"=w1094, "deviceId"=w1083) -> ("measurementData"=w1101:T8[])  [unwired: 4 in, 4 out]
            n92 = Open/Create/Replace File(file path (use dialog)=w1087, operation (0:open)=T6."replace or create with confirmation") -> (refnum out=w1100:refnum<file>, error out=w1097:errorcluster)  [unwired: 4 in, 1 out]
            n93 = for {
              tunnel: w1101 -> [w1118] mode=indexing
              tunnel: w1100 -> [w1107]
              tunnel: [w1105] -> w1099
              tunnel: w1097 -> [w1104]
              tunnel: [w1103] -> w1096
              n94 = Unbundle By Name(w1118) -> ("outMeasurementData"=w1116:T9[])
              n95 = Index Array(array=w1116, index=0) -> (element=w1115:T9)
              n96 = Unbundle By Name(w1115) -> ("measurementValue"=w1112:i32)
              n97 = To Double Precision Float(number=w1112) -> (double precision float=w1113:dbl)
              n98 = Divide(x=w1113, y=1000.0) -> (x/y=w1111:dbl)
              n99 = Format Into String(format string="%.6f%s", error in=w1104, w1111, "\r\n") -> (resulting string=w1108:string, error out=w1106:errorcluster)  [unwired: 1 in]
              n100 = Write to Text File(file (use dialog)=w1107, text=w1108, error in=w1106) -> (refnum out=w1105:refnum<file>, error out=w1103:errorcluster)  [unwired: 1 in, 1 out]
            }
            n101 = Close File(refnum=w1099, error in=w1096) -> (error out=w1079:errorcluster)  [unwired: 1 out]
            n102 = call <vilib>:"Clear Errors.vi"("error in (no error)"=w1079, "specific error code to clear (0: all)"=43) -> ("error out"=w1078:errorcluster)  [unwired: 4 in, 1 out]
            n103 = Merge Errors(w1078, w1081) -> (w1082:errorcluster)
          }
          frame "Check Time" {
            n104 = case shown="True" w1119 {
              tunnel: w1122 -> [_ w1129]
              tunnel: [w1127 w1128] -> w1121
              frame False {
                w1127 = Sensor_Station_States."Close"  # Next State
                # "Close Chromatic Connection"
              }
              frame True {
                w1130 = Sensor_Station_States."Acquire"  # Next State
                # "Wait Until Target Time Elapsed"
                n105 = Select(t=w1130, s=w1129, f=Sensor_Station_States."Check Time" ("Next State")) -> (s? t:f=w1128:T5)
              }
            }
            n106 = Wait (ms)(milliseconds to wait=u32 10) -> ()  [unwired: 1 out]
          }
          frame "Close" {
            w1137 = Sensor_Station_States."Close"  # Not Used
            n107 = case shown="True" w1134 {
              tunnel: w1141 -> [_ w1143]
              frame False {
              }
              frame True {
                n108 = local read "Device ID"() -> (w1142:i32)
                n109 = call "Close.vi"("error in (no error)"=w1143, "deviceId"=w1142) -> ()  [unwired: 9 in, 1 out]
              }
            }
            n110 = local read "STOP"() -> (w1132:bool)
            n111 = Select(t=w1137, s=w1132, f=Sensor_Station_States."Idle" ("Next State")) -> (s? t:f=w1135:T5)
          }
        }
        "Chromatic Sensor Error" <- w955
        n112 = local read "STOP"() -> (w956:bool)
        n113 = Select(t=Sensor_Station_States."Close" ("Next State"), s=w956, f=w962) -> (s? t:f=w960:T5)
      }
      n114 = while {
        shift-right: [w51] -> _
        shift-left: w11 -> [w63]
        shift-right: [w59] -> _
        shift-left: TRUE -> [w61]
        shift-right: [w57] -> _
        shift-left: w13 -> [w58]
        shift-right: [w44] -> _
        shift-left: _ -> [w56]
        shift-right: [w55] -> _
        shift-left: w10 -> [w54]
        shift-right: [w47] -> _
        shift-left: w9 -> [w46]
        shift-right: [w42] -> _
        shift-left: refnum<vi> refnum ("application reference") -> [w41]
        shift-right: [w43] -> _
        shift-left: refnum<vi> refnum -> [w40]
        stop <- w50 stop-if-true
        w62 = 0.05  # target time
        n115 = call "Elapsed Time2"("Time Target (s)"=w62, "Reset"=w61) -> ("Time has Elapsed"=w60:bool)  [unwired: 10 in, 7 out]
        n116 = case shown="\"Save\"" w63 {
          tunnel: w56 -> [w70 w108 w121 w127 w140 w182 w194 w215]
          tunnel: [w75 w98 Sensor_Station_States."Log" ("Next State") w133 w161 w179 w199 w217] -> w53
          tunnel: w60 -> [_ _ _ _ _ w180 _ _]
          tunnel: [_ w109 _ _ _ _ _ _] -> w59
          tunnel: w58 -> [w74 w106 w120 w129 w158 w184 _ w213]
          tunnel: [w74 w106 w120 w129 w158 w184 FALSE ("Chromatic Logging?") w213] -> w57
          tunnel: [w69 w103 w121 w125 w148 w182 errorcluster {"status"=FALSE, "code"=0, "source"=""} ("error constant") w215] -> w44
          tunnel: [w66 w107 w122 w135 w159 w183 FALSE w214] -> w55
          tunnel: w54 -> [_ w107 w122 w135 w159 w183 w191 w214]
          tunnel: [_ _ _ _ _ _ w197 _] -> w50
          tunnel: "Enable Laser" -> [w73 _ _ _ _ w181 _ w218]
          tunnel: [w71 w105 w112 w130 w160 w178 0.0 w212] -> w47
          tunnel: w46 -> [w71 _ w112 w130 w160 w178 _ w212]
          tunnel: "Laser Data\nLogging" -> [_ _ _ w131 _ _ _ _]
          tunnel: [w68 w95 w110 w123 w145 w176 refnum<vi> refnum w210] -> w43
          tunnel: [w67 w96 w111 w124 w146 w177 refnum<vi> refnum ("application reference") w211] -> w42
          tunnel: w41 -> [w65 w96 w111 w124 w146 w177 w196 w211]
          tunnel: w40 -> [w64 w95 w110 w123 w145 w176 w195 w210]
          frame "Initialise", Default {
            w72 = Sensor_Station_States."Acquire"  # Next State
            n117 = case shown="True" w73 {
              tunnel: [FALSE w85] -> w66
              tunnel: w70 -> [w79 w84]
              tunnel: [w79 w81] -> w69
              tunnel: [w78 w88] -> w67
              tunnel: [w77 w87] -> w68
              tunnel: w65 -> [w78 _]
              tunnel: w64 -> [w77 _]
              frame False {
              }
              frame True {
                # "Set cRIO Variable to default"
                n118 = Open Application Reference(8:w84, 11:"NI-cRIO-9066-TCD" ("machine name (\"\":  open local reference)")) -> (0:w92:errorcluster, 3:w88:refnum<vi>)  [unwired: 2 in]
                n119 = Open VI Reference(application reference (local)=w88, vi path=path "/home/lvuser/natinst/bin/cRIO_triggered_laser_log.vi", error in (no error)=w92) -> (vi reference=w87:refnum<vi>, error out=w91:errorcluster)  [unwired: 3 in]
                n120 = shared-variable "NI-cRIO-9066-TCD\\cRioLibrary.lvlib\\cRioTransferData"(FALSE ("cRioTransferData")) -> (error out=w82:errorcluster)  [unwired: 1 in]
                n121 = invoke class="VI" method="Run VI"(reference=w87, error in=w91, "Wait until done"=FALSE ("Wait Until Done")) -> (error out=w83:errorcluster)  [unwired: 2 in, 4 out]
                n122 = Merge Errors(w83, w82) -> (w81:errorcluster)
                n123 = Unbundle By Name(w83) -> ("status"=w86:bool)
                n124 = Not(x=w86) -> (.not. x?=w85:bool)
              }
            }
            n125 = local write "Enable Laser"(w66) -> ()
            n126 = Select(t=w72, s=w66, f=Sensor_Station_States."Idle" ("Next State")) -> (s? t:f=w75:T5)
          }
          frame "Acquire" {
            w109 = TRUE  # Reset Elapsed Time counter
            # "Next State"
            # "Laser output connected \nto cRIO module AI1"
            n127 = shared-variable "NI-cRIO-9066-TCD\\Mod3\\AI1"(error in=w108) -> (w105:dbl, error out=w101:errorcluster)
            n128 = Unbundle By Name(w101) -> ("status"=w102:bool)
            n129 = call <vilib>:"Simple Error Handler.vi"("error in (no error)"=w101) -> ("error out"=w104:errorcluster)  [unwired: 4 in, 4 out]
            n130 = Not(x=w102) -> (.not. x?=w100:bool)
            n131 = local write "Enable Laser"(w100) -> ()
            n132 = call <vilib>:"Clear Errors.vi"("error in (no error)"=w104) -> ("error out"=w103:errorcluster)  [unwired: 5 in, 1 out]
            n133 = Select(t=Sensor_Station_States."Visualise" ("Next State"), s=w100, f=Sensor_Station_States."Idle" ("Next State")) -> (s? t:f=w98:T5)
          }
          frame "Visualise" {
            # "Next State"
            # "Convert to um"
            # "Convert 0-5V to distance (mm)"
            n134 = Multiply(x=w112, y=2.0) -> (x*y=w117:dbl)
            n135 = Subtract(x=w117, y=5.0) -> (x-y=w115:dbl)
            n136 = Multiply(x=1000.0, y=w115) -> (x*y=→"Laser Displacement (cRIO)":dbl)
          }
          frame "Log" {
            # "Transfer once data file has\nbeen created"
            # "Next State"
            # "Trigger cRIO to start / stop \nlogging data"
            n137 = shared-variable "NI-cRIO-9066-TCD\\cRioLibrary.lvlib\\logData"(w131, error in=w127) -> (error out=w126:errorcluster)
            n138 = shared-variable "NI-cRIO-9066-TCD\\cRioLibrary.lvlib\\cRioTransferData"(error in=w126) -> (w128:bool, error out=w125:errorcluster)
            n139 = Select(t=Sensor_Station_States."Save" ("Next State"), s=w128, f=Sensor_Station_States."Check Time" ("Next State")) -> (s? t:f=w133:T5)
          }
          frame "Save" {
            w161 = Sensor_Station_States."Check Time"  # Next State
            n140 = local read "Save Directory"() -> (w157:path)
            n141 = local read "Test Name"() -> (w149:string)
            n142 = local read "Suffix"() -> (w150:string)
            n143 = Path To String(path=w157) -> (string=w156:string)
            n144 = Concatenate Strings(w156, "\\" ("string"), w149, w150, "_laser.csv" ("string")) -> (w154:string)
            n145 = String To Path(string=w154) -> (path=w153:path)
            n146 = Open/Create/Replace File(file path (use dialog)=w153, error in=w140, operation (0:open)=T6."replace or create with confirmation", disable buffering (F)=TRUE) -> (refnum out=w144:refnum<file>, cancelled=w139:bool, error out=w141:errorcluster)  [unwired: 2 in]
            n147 = case shown="False" w139 {
              tunnel: w144 -> [w162 w174]
              tunnel: [w167 w175] -> w143
              tunnel: w141 -> [w166 w175]
              tunnel: [w162 w174] -> w138
              frame False {
                # "Access cRIO PC"
                # "Logged data location on cRIO"
                n148 = call <vilib>:"Open Session.vi"("host uri prefix"="http://NI-cRIO-9066-TCD/files", "username"="admin", "password"="", "error in (no error)"=w166) -> ("session handle out"=w170:T14, "error out"=w165:errorcluster)  [unwired: 10 in]
                n149 = Refnum to Path(1:w162) -> (0:w164:path)
                n150 = call-poly <vilib>:"Get.vi"("session handle"=w170, "relative uri"="/home/lvuser/cRIO_logged_data.csv", "local file path"=w164, "error in (no error)"=w165) -> ("session handle out"=w169:T14, "error out"=w168:errorcluster)  [unwired: 9 in, 1 out]
                n151 = call <vilib>:"Close Session.vi"("session handle"=w169, "error in (no error)"=w168) -> ("error out"=w167:errorcluster)  [unwired: 13 in]
              }
              frame True {
              }
            }
            n152 = shared-variable "NI-cRIO-9066-TCD\\cRioLibrary.lvlib\\cRioTransferData"(FALSE ("cRioTransferData")) -> ()  [unwired: 1 in, 1 out]
            n153 = Close File(refnum=w138, error in=w143) -> (error out=w142:errorcluster)  [unwired: 1 out]
            n154 = call <vilib>:"Clear Errors.vi"("error in (no error)"=w142, "specific error code to clear (0: all)"=43) -> ("error out"=w148:errorcluster)  [unwired: 4 in, 1 out]
          }
          frame "Check Time" {
            n155 = case shown="False" w181 {
              tunnel: w180 -> [_ w188]
              tunnel: [w186 w187] -> w179
              frame False {
                w186 = Sensor_Station_States."Close"  # Next State
                # "Close Laser Connection"
              }
              frame True {
                w189 = Sensor_Station_States."Acquire"  # Next State
                # "Wait Until Target Time Elapsed"
                n156 = Select(t=w189, s=w188, f=Sensor_Station_States."Check Time" ("Next State")) -> (s? t:f=w187:T5)
              }
            }
            n157 = Wait (ms)(milliseconds to wait=u32 20) -> ()  [unwired: 1 out]
          }
          frame "Close" {
            w200 = Sensor_Station_States."Close"  # Not Used
            n158 = case shown="True" w191 {
              tunnel: w196 -> [_ w208]
              tunnel: w195 -> [_ w207]
              tunnel: w194 -> [_ w206]
              frame False {
              }
              frame True {
                n159 = Close Reference(reference=w207, error in (no error)=w206) -> (error out=w209:errorcluster)
                n160 = Close Reference(reference=w208, error in (no error)=w209) -> (error out=w205:errorcluster)
                n161 = call <vilib>:"Simple Error Handler.vi"("error in (no error)"=w205) -> ()  [unwired: 4 in, 5 out]
              }
            }
            n162 = local read "STOP"() -> (w197:bool)
            n163 = Select(t=w200, s=w197, f=Sensor_Station_States."Idle" ("Next State")) -> (s? t:f=w199:T5)
          }
          frame "Idle" {
            # "Next State"
            n164 = Wait (ms)(milliseconds to wait=u32 200) -> ()  [unwired: 1 out]
            n165 = Select(t=Sensor_Station_States."Initialise" ("Next State"), s=w218, f=Sensor_Station_States."Idle" ("Next State")) -> (s? t:f=w217:T5)
          }
        }
        "Laser Sensor Error" <- w44
        n166 = local read "STOP"() -> (w49:bool)
        n167 = Select(t=Sensor_Station_States."Close" ("Next State"), s=w49, f=w53) -> (s? t:f=w51:T5)
      }
      n168 = while {
        tunnel: "Connection?" -> [w244]
        tunnel: [w241] -> w38
        tunnel: [w231] -> w37
        shift-right: [w234] -> _
        shift-left: w36 -> [w237]
        tunnel: w36 -> [w233]
        tunnel: w35 -> [w230]
        tunnel: [w229] -> w34
        shift-right: [w226] -> _
        shift-left: w15 -> [w225]
        shift-right: [w223] -> _
        shift-left: w14 -> [w224]
        stop <- "STOP" stop-if-true
        n169 = invoke class="TrioPC" method="IsOpen"(reference=w244, "lMode"=-1) -> (reference out=w228:refnum<k7>, error out=w227:errorcluster, "IsOpen"=w242:bool)  [unwired: 2 in, 1 out]
        "IsOpen" <- w242
        n170 = Tick Count (ms)() -> (millisecond timer value=w234:u32)
        n171 = Wait Until Next ms Multiple(millisecond multiple=u32 40) -> ()  [unwired: 1 out]
        n172 = Subtract(x=w234, y=w233) -> (x-y=w232:u32)
        n173 = Subtract(x=w234, y=w237) -> (x-y=→"Loop Time (us)":u32)
        n174 = case shown="True" "Connect  to Controller" {
          tunnel: [w250 w284] -> w241
          tunnel: [w251 w283] -> w231
          tunnel: w242 -> [w247 w282]
          tunnel: w228 -> [w249 w281]
          tunnel: w227 -> [w248 w280]
          tunnel: w230 -> [_ w279]
          tunnel: [_ w278] -> w229
          tunnel: [_ w277] -> w226
          tunnel: w225 -> [_ w276]
          tunnel: w224 -> [_ w275]
          tunnel: [_ w274] -> w223
          frame False {
            n175 = case shown="True" w247 {
              tunnel: [w258 w263] -> w253
              tunnel: [w257 w262] -> w252
              tunnel: w249 -> [w258 w260]
              tunnel: w248 -> [w257 w259]
              frame False {
              }
              frame True {
                n176 = invoke class="TrioPC" method="Close"(reference=w260, error in=w259) -> (reference out=w263:refnum<k7>, error out=w262:errorcluster)  [unwired: 2 in, 2 out]
                n177 = property on="Set Parameters" class="Bool"("Disabled"=u8 0) -> ()  [unwired: 2 in, 2 out]
              }
            }
            n178 = local read "Controller Connection Type"() -> (w246:string)
            n179 = Select(t=w246, s="Set Parameters", f="") -> (s? t:f=w254:string)
            n180 = case shown="\"1\"" w254 {
              tunnel: w253 -> [w265 w268 w273]
              tunnel: w252 -> [w264 w267 w272]
              tunnel: [w265 w270 w273] -> w250
              tunnel: [w264 w269 w272] -> w251
              frame "", Default {
              }
              frame "2" {
                # "Ethernet"
                n181 = call "SubEthernetSettings.vi"() -> ("Ethernet IP Address 2"=w266:string)
                n182 = property class="TrioPC"(reference=w268, error in=w267, "HostAddress"=w266) -> (reference out=w270:refnum<k7>, error out=w269:errorcluster)
              }
              frame "1" {
                # "Serial"
                n183 = call "SubSerialSettings.vi"() -> ("CommPort"=→"Serial Port":fxp<+,3,3>)
              }
            }
          }
          frame True {
            # "Open State"
            n184 = case shown="True" w282 {
              tunnel: [w288 w372] -> w284
              tunnel: [w289 w365] -> w283
              tunnel: w281 -> [w293 w338]
              tunnel: w280 -> [w292 w343]
              tunnel: w279 -> [_ w382]
              tunnel: [_ w381] -> w278
              tunnel: [_ w379] -> w277
              tunnel: w276 -> [_ w378]
              tunnel: w275 -> [_ w377]
              tunnel: [_ w376] -> w274
              frame False {
                # "Connecting State"
                n185 = Decimal String To Number(string="Controller Connection Type") -> (number=w290:i32)  [unwired: 2 in, 1 out]
                n186 = case shown="2" w290 {
                  tunnel: [i16 0 ("PortId") w329 i16 3240 ("PortId")] -> w297
                  frame 0, Default {
                  }
                  frame 1 {
                    n187 = local read "Serial Port"() -> (w329:fxp<+,3,3>)
                  }
                  frame 2 {
                  }
                }
                n188 = invoke class="TrioPC" method="Open"(reference=w293, error in=w292, "PortType"=w290, "PortId"=w297) -> (reference out=w287:refnum<k7>, error out=w286:errorcluster, "Open"=w285:bool)  [unwired: 1 in, 2 out]
                n189 = local write "Connect  to Controller"(w285) -> ()
                n190 = Select(t=u8 2, s=w285, f=u8 0 ("Disabled")) -> (s? t:f=w294:u8)
                n191 = property on="Set Parameters" class="Bool"("Disabled"=w294) -> ()  [unwired: 2 in, 2 out]
                n192 = case shown="False" w285 {
                  tunnel: [w299 w325] -> w289
                  tunnel: [w300 w324] -> w288
                  tunnel: w287 -> [w300 w315]
                  tunnel: w286 -> [w299 w306]
                  frame False {
                    n193 = One Button Dialog(message="Controller Not Found\nPlease check connection") -> ()  [unwired: 1 in, 1 out]
                  }
                  frame True {
                    # "Programs on Controller to be excluded from drop down menu"
                    n194 = invoke class="TrioPC" method="GetVariable"(reference=w315, error in=w306, "Variable"="CONTROL") -> (reference out=w308:refnum<k7>, error out=w307:errorcluster, "Value"=w312:dbl)  [unwired: 2 in, 2 out]
                    n195 = Number To Decimal String(number=w312) -> (decimal integer string=→"Controller Type":string)  [unwired: 1 in]
                    n196 = invoke class="TrioPC" method="GetVariable"(reference=w308, error in=w307, "Variable"="VERSION") -> (reference out=w304:refnum<k7>, error out=w305:errorcluster, "Value"=w311:dbl)  [unwired: 2 in, 2 out]
                    n197 = Number To Decimal String(number=w311) -> (decimal integer string=→"Version":string)  [unwired: 1 in]
                    n198 = invoke class="TrioPC" method="ProductName"(reference=w304, error in=w305) -> (reference out=w303:refnum<k7>, error out=w302:errorcluster, "ProductName"=→"Product Name":string)  [unwired: 1 in]
                    n199 = invoke class="TrioPC" method="Dir"(reference=w303, error in=w302) -> (reference out=w324:refnum<k7>, error out=w325:errorcluster, "Directory"=w326:string)  [unwired: 3 in, 2 out]
                    n200 = Initialize Array("BLA" ("element")) -> (w323:string[])  [unwired: 1 in]
                    n201 = Insert Into Array(array=w323, new element #1="MC_CONFIG" ("element"), new element #2="PROJECT_DATA" ("element"), new element #3="CAMLIB.CAM" ("element"), new element #4="IEC" ("element"), new element #5="HMIDESIGN.HMI") -> (w316:string[])  [unwired: 1 in]
                    n202 = call "Controller - Get Programs (subVI).vi"("Controller Directory"=w326, "Exclusion List"=w316) -> ("Programs List"=w327:string[])
                    n203 = property on="Select Program" class="CmbBox"("Strings[]"=w327) -> ()  [unwired: 2 in, 2 out]
                  }
                }
              }
              frame True {
                # "Connected"
                n204 = Build Array("MSPEED", "ENDMOVE", "MPOS") -> (w344:string[])
                n205 = call "Controller - Get Axis Parameters (subVI).vi"("Axis"=i16 0, "Axis Parameters"=w344, "error in (no error)"=w343, "Automation Refnum in"=w338) -> ("Axis Parameter Values"=w345:dbl[], "error out"=w342:errorcluster)  [unwired: 5 in, 1 out]
                n206 = call "Controller - Get Axis Parameters (subVI).vi"("Axis"=i16 1, "Axis Parameters"=w344, "Automation Refnum in"=w338) -> ("Axis Parameter Values"=w346:dbl[], "error out"=w341:errorcluster)  [unwired: 6 in, 1 out]
                n207 = call "Controller - Get Axis Parameters (subVI).vi"("Axis"=i16 2, "Axis Parameters"=w344, "Automation Refnum in"=w338) -> ("Axis Parameter Values"=w347:dbl[], "error out"=w340:errorcluster)  [unwired: 6 in, 1 out]
                n208 = Merge Errors(w342, w341, w340) -> (w339:errorcluster)
                n209 = case shown="\"MONITORING\"" "Setup Tab" {
                  tunnel: w338 -> [w400 w431]
                  tunnel: [w399 w431] -> w337
                  tunnel: [w396 w430] -> w363
                  tunnel: [w383 w435] -> w362
                  tunnel: [w384 w436] -> w355
                  tunnel: w347 -> [_ w434]
                  tunnel: w346 -> [w385 w433]
                  tunnel: w345 -> [w386 w432]
                  tunnel: w339 -> [w395 w430]
                  frame "SETUP", Default {
                    n210 = call "Is Value Changed.vim"("value"="Axis Enable") -> ("changed or first call?"=w402:bool)
                    n211 = Index Array(array=w386) -> (element #2=w391:dbl, element #3=w392:dbl)  [unwired: 3 in, 1 out]
                    n212 = Index Array(array=w385) -> (element #2=w394:dbl, element #3=w393:dbl)  [unwired: 3 in, 1 out]
                    n213 = case shown="True" w402 {
                      tunnel: [w412 w417] -> w398
                      tunnel: w395 -> [w412 w414]
                      tunnel: w400 -> [w411 w416]
                      tunnel: "Axis Enable" -> [_ w415]
                      tunnel: [w411 w413] -> w399
                      frame False {
                      }
                      frame True {
                        n214 = case shown="False" w415 {
                          tunnel: [w419 w425] -> w417
                          tunnel: w414 -> [w420 w426]
                          tunnel: w416 -> [w421 w427]
                          tunnel: [w418 w424] -> w413
                          frame False {
                            n215 = invoke class="TrioPC" method="SetVariable"(reference=w421, error in=w420, "Variable"="WDOG", "Value"=0.0) -> (reference out=w418:refnum<k7>, error out=w419:errorcluster)  [unwired: 1 in, 3 out]
                          }
                          frame True {
                            n216 = invoke class="TrioPC" method="SetVariable"(reference=w427, error in=w426, "Variable"="WDOG", "Value"=1.0) -> (reference out=w424:refnum<k7>, error out=w425:errorcluster)  [unwired: 1 in, 3 out]
                          }
                        }
                      }
                    }
                    n217 = case shown="True" "Home Axes" {
                      tunnel: w400 -> [w405 w409]
                      tunnel: w395 -> [w404 w408]
                      tunnel: [w405 w407] -> _
                      tunnel: [w404 w406] -> w397
                      frame False {
                      }
                      frame True {
                        n218 = invoke class="TrioPC" method="Run"(reference=w409, error in=w408, "Program"="HOME_ALL") -> (reference out=w407:refnum<k7>, error out=w406:errorcluster)  [unwired: 2 in, 3 out]
                      }
                    }
                    n219 = Absolute Value(x=w394) -> (abs(x)=w389:dbl)
                    n220 = Absolute Value(x=w391) -> (abs(x)=w387:dbl)
                    n221 = Absolute Value(x=w393) -> (abs(x)=w390:dbl)
                    n222 = Absolute Value(x=w392) -> (abs(x)=w388:dbl)
                    n223 = Subtract(x=w389, y=w390) -> (x-y=w383:dbl)
                    n224 = Subtract(x=w387, y=w388) -> (x-y=w384:dbl)
                    n225 = Merge Errors(w398, w397) -> (w396:errorcluster)
                  }
                  frame "MONITORING" {
                    n226 = Index Array(array=w432) -> (element #1=→"Axis 0 Velocity":dbl, element #2=w454:dbl, element #3=w455:dbl)  [unwired: 3 in]
                    "Axis 0 Position" <- w455
                    "Axis 0 End Pos" <- w454
                    n227 = Index Array(array=w433) -> (element #1=→"Axis 1 Velocity":dbl, element #2=w458:dbl, element #3=w457:dbl)  [unwired: 3 in]
                    "Axis 1 Position" <- w457
                    "Axis 1 End Pos" <- w458
                    n228 = Index Array(array=w434) -> (element #1=→"Axis 2 Velocity":dbl, element #2=w438:dbl, element #3=w437:dbl)  [unwired: 3 in]
                    "Axis 2 Position" <- w437
                    "Axis 2 End Pos" <- w438
                    n229 = Delete From Array(array=w432, length=1, index=0) -> (array with subset deleted=w447:dbl[])  [unwired: 1 out]
                    n230 = Delete From Array(array=w433, length=1, index=0) -> (array with subset deleted=w446:dbl[])  [unwired: 1 out]
                    n231 = Absolute Value(x=w438) -> (abs(x)=w440:dbl)
                    n232 = Absolute Value(x=w454) -> (abs(x)=w449:dbl)
                    n233 = Absolute Value(x=w458) -> (abs(x)=w451:dbl)
                    n234 = Absolute Value(x=w437) -> (abs(x)=w439:dbl)
                    n235 = Absolute Value(x=w455) -> (abs(x)=w450:dbl)
                    n236 = Absolute Value(x=w457) -> (abs(x)=w452:dbl)
                    n237 = Build Cluster Array(w447, w446) -> (→"XY Graph":cluster{dbl, dbl}[])
                    n238 = Subtract(x=w440, y=w439) -> (x-y=→"A2 Remaining":dbl)
                    n239 = Subtract(x=w449, y=w450) -> (x-y=w436:dbl)
                    "A0 Remaining" <- w436
                    n240 = Subtract(x=w451, y=w452) -> (x-y=w435:dbl)
                    "A1 Remaining" <- w435
                  }
                }
                n241 = call "Is Value Changed.vim"("value"="Motion Tab") -> ("changed or first call?"=w331:bool)
                n242 = case shown="\"POSITION\", Default" "Motion Tab" {
                  tunnel: w363 -> [w464 w709]
                  tunnel: [w473 w706] -> w373
                  tunnel: w337 -> [w465 w710]
                  tunnel: [w470 w711] -> w336
                  tunnel: w382 -> [w469 _]
                  tunnel: [w474 _] -> w381
                  tunnel: "Measurement\nAxis" -> [_ w701]
                  tunnel: [_ w716] -> w379
                  tunnel: w378 -> [_ w715]
                  tunnel: w377 -> [_ w714]
                  tunnel: [_ w713] -> w376
                  tunnel: w355 -> [_ w708]
                  tunnel: w362 -> [_ w707]
                  tunnel: w331 -> [w467 _]
                  frame "POSITION", Default {
                    n243 = case shown="True" "Run Program" {
                      tunnel: w464 -> [w479 w484]
                      tunnel: [w479 w483] -> w462
                      tunnel: w465 -> [w478 w482]
                      tunnel: [w478 w481] -> w463
                      frame False {
                      }
                      frame True {
                        n244 = invoke class="TrioPC" method="Run"(reference=w482, error in=w484, "Program"="Select Program") -> (reference out=w481:refnum<k7>, error out=w483:errorcluster)  [unwired: 2 in, 3 out]
                      }
                    }
                    n245 = call "Is Value Changed.vim"("value"="Run Program") -> ("changed or first call?"=w460:bool)
                    n246 = case shown="False" "Set Parameters 2" {
                      tunnel: [w601 w644] -> w476
                      tunnel: w465 -> [w604 w639]
                      tunnel: w464 -> [w603 w638]
                      tunnel: [w602 w637] -> w477
                      tunnel: w467 -> [w600 _]
                      tunnel: w460 -> [w599 _]
                      frame False {
                        n247 = Or(x=w600, y=w599) -> (x .or. y?=w598:bool)
                        n248 = case shown="True" w598 {
                          tunnel: w604 -> [w606 w623]
                          tunnel: w603 -> [w605 w620]
                          tunnel: [w606 w622] -> w602
                          tunnel: [w605 w621] -> w601
                          frame False {
                          }
                          frame True {
                            n249 = Build Array("SPEED", "ACCEL", "JOGSPEED") -> (w624:string[])
                            n250 = for {
                              N: 3 -> [_]
                              tunnel: w624 -> [w636]
                              tunnel: w623 -> [w635]
                              tunnel: [w632] -> w619 mode=indexing
                              tunnel: [w631] -> w622
                              shift-right: [w630] -> w621
                              shift-left: w620 -> [w629]
                              i -> [w634]
                              n251 = To Word Integer(number=w634) -> (16bit integer=w633:i16)
                              n252 = call "Controller - Get Axis Parameters (subVI).vi"("Axis"=w633, "Axis Parameters"=w636, "error in (no error)"=w629, "Automation Refnum in"=w635) -> ("Axis Parameter Values"=w632:dbl[], "error out"=w630:errorcluster, "Automation Refnum out"=w631:refnum<k7>)  [unwired: 5 in]
                            }
                            n253 = Index Array(array=w619) -> (element #1=w618:dbl[], element #2=w617:dbl[], element #3=w616:dbl[])  [unwired: 6 in]
                            n254 = Index Array(array=w618) -> (element #1=w615:dbl, element #2=w614:dbl, element #3=w613:dbl)  [unwired: 3 in]
                            n255 = Index Array(array=w617) -> (element #1=w611:dbl, element #2=w612:dbl, element #3=w610:dbl)  [unwired: 3 in]
                            n256 = Index Array(array=w616) -> (element #1=w608:dbl, element #2=w609:dbl, element #3=w607:dbl)  [unwired: 3 in]
                            n257 = local write "Axis 0 Speed"(w615) -> ()
                            n258 = local write "Axis 0 Acc"(w614) -> ()
                            n259 = local write "Axis 0 Jogspeed"(w613) -> ()
                            n260 = local write "Axis 1 Speed"(w611) -> ()
                            n261 = local write "Axis 1 Acc"(w612) -> ()
                            n262 = local write "Axis 1 Jogspeed"(w610) -> ()
                            n263 = local write "Axis 2 Speed"(w608) -> ()
                            n264 = local write "Axis 2 Acc"(w609) -> ()
                            n265 = local write "Axis 2 Jogspeed"(w607) -> ()
                          }
                        }
                      }
                      frame True {
                        n266 = Build Array("Axis 0 Speed", "Axis 1 Speed", "Axis 2 Speed") -> (w650:dbl[])
                        n267 = Build Array("Axis 0 Acc", "Axis 1 Acc", "Axis 2 Acc") -> (w649:dbl[])
                        n268 = Build Array("Axis 0 Jogspeed", "Axis 1 Jogspeed", "Axis 2 Jogspeed") -> (w640:dbl[])
                        n269 = for {
                          N: 3 -> [_]
                          tunnel: w650 -> [w662] mode=indexing
                          tunnel: w649 -> [w661] mode=indexing
                          tunnel: w640 -> [w663] mode=indexing
                          shift-right: [w654] -> w644
                          shift-left: w638 -> [w658]
                          shift-right: [w655] -> w637
                          shift-left: w639 -> [w659]
                          i -> [w660]
                          n270 = invoke class="TrioPC" method="SetAxisVariable"(reference=w659, error in=w658, "Variable"="SPEED", "Axis"=w660, "Value"=w662) -> (reference out=w670:refnum<k7>, error out=w669:errorcluster)  [unwired: 1 in, 4 out]
                          n271 = invoke class="TrioPC" method="SetAxisVariable"(reference=w670, error in=w669, "Variable"="ACCEL", "Axis"=w660, "Value"=w661) -> (reference out=w668:refnum<k7>, error out=w667:errorcluster)  [unwired: 1 in, 4 out]
                          n272 = invoke class="TrioPC" method="SetAxisVariable"(reference=w668, error in=w667, "Variable"="DECEL", "Axis"=w660, "Value"=w661) -> (reference out=w657:refnum<k7>, error out=w656:errorcluster)  [unwired: 1 in, 4 out]
                          n273 = invoke class="TrioPC" method="SetAxisVariable"(reference=w657, error in=w656, "Variable"="JOGSPEED", "Axis"=w660, "Value"=w663) -> (reference out=w655:refnum<k7>, error out=w654:errorcluster)  [unwired: 1 in, 4 out]
                        }
                      }
                    }
                    n274 = case shown="True" "Jog Axes" {
                      selector: "Jog Axes" -> [w490 _]
                      tunnel: w469 -> [w491 w502]
                      tunnel: [w491 w501] -> w474
                      tunnel: w463 -> [w488 w504]
                      tunnel: w462 -> [w487 w503]
                      tunnel: [w486 w499] -> w466
                      tunnel: [w485 w500] -> _
                      frame False {
                        n275 = call "Is Value Changed.vim"("value"=w490) -> ("changed or first call?"=w489:bool)
                        n276 = case shown="True" w489 {
                          tunnel: [w493 w497] -> w485
                          tunnel: [w492 w496] -> w486
                          tunnel: w488 -> [w493 w495]
                          tunnel: w487 -> [w492 w494]
                          frame False {
                          }
                          frame True {
                            n277 = invoke class="TrioPC" method="Execute"(reference=w495, error in=w494, "Command"="OP(50,55,OFF)") -> (reference out=w497:refnum<k7>, error out=w496:errorcluster)  [unwired: 1 in, 2 out]
                          }
                        }
                      }
                      frame True {
                        w511 = 0 ("f")
                        n278 = Select(t=1, s="Up Button", f=w511) -> (s? t:f=w518:i32)
                        n279 = Select(t=2, s="Down Button", f=w511) -> (s? t:f=w517:i32)
                        n280 = Select(t=3, s="Previous Button", f=w511) -> (s? t:f=w516:i32)
                        n281 = Select(t=4, s="Next Button", f=w511) -> (s? t:f=w515:i32)
                        n282 = Select(t=5, s="Top Button", f=w511) -> (s? t:f=w514:i32)
                        n283 = Select(t=6, s="Bottom Button", f=w511) -> (s? t:f=w513:i32)
                        n284 = Compound Arithmetic op=ADD(w518, w517, w516, w515, w514, w513) -> (w512:i32)
                        n285 = case shown="0, Default" w512 {
                          tunnel: w504 -> [w530 w571 w577 w581 w587 w592 w597]
                          tunnel: w503 -> [w529 w570 w576 w582 w586 w591 w596]
                          tunnel: [w528 w568 w575 w580 w585 w590 w595] -> w500
                          tunnel: [w527 w569 w574 w579 w584 w589 w594] -> w499
                          tunnel: w502 -> [w526 _ _ _ _ _ _]
                          tunnel: [w525 _ _ _ _ _ _] -> w501
                          frame 0, Default {
                            n286 = call-poly <vilib>:"Acquire Input Data.vi"("device ID"=w526) -> ("device ID"=w525:refnum<k1>, "keys pressed"=w531:T15)  [unwired: 1 in, 16 out]
                            n287 = Index Array(array=w531) -> (element=w532:T2)  [unwired: 1 in]
                            "1st Key" <- w532
                            n288 = case shown="\"0\", Default" w532 {
                              tunnel: w530 -> [w537 w541 w547 w551 w557 w562 w567]
                              tunnel: w529 -> [w536 w542 w546 w550 w556 w561 w566]
                              tunnel: [w535 w540 w545 w548 w555 w560 w565] -> w528
                              tunnel: [w534 w539 w544 w549 w554 w559 w564] -> w527
                              frame "0", Default {
                                n289 = invoke class="TrioPC" method="Execute"(reference=w537, error in=w536, "Command"="OP(50,55,OFF)") -> (reference out=w535:refnum<k7>, error out=w534:errorcluster)  [unwired: 1 in, 2 out]
                              }
                              frame "LEFT" {
                                n290 = invoke class="TrioPC" method="Execute"(reference=w541, error in=w542, "Command"="OP(50,ON)") -> (reference out=w540:refnum<k7>, error out=w539:errorcluster)  [unwired: 1 in, 2 out]
                              }
                              frame "RIGHT" {
                                n291 = invoke class="TrioPC" method="Execute"(reference=w547, error in=w546, "Command"="OP(51,ON)") -> (reference out=w545:refnum<k7>, error out=w544:errorcluster)  [unwired: 1 in, 2 out]
                              }
                              frame "UP" {
                                n292 = invoke class="TrioPC" method="Execute"(reference=w551, error in=w550, "Command"="OP(53,ON)") -> (reference out=w548:refnum<k7>, error out=w549:errorcluster)  [unwired: 1 in, 2 out]
                              }
                              frame "DOWN" {
                                n293 = invoke class="TrioPC" method="Execute"(reference=w557, error in=w556, "Command"="OP(52,ON)") -> (reference out=w555:refnum<k7>, error out=w554:errorcluster)  [unwired: 1 in, 2 out]
                              }
                              frame "PRIOR (PG UP)" {
                                n294 = invoke class="TrioPC" method="Execute"(reference=w562, error in=w561, "Command"="OP(54,ON)") -> (reference out=w560:refnum<k7>, error out=w559:errorcluster)  [unwired: 1 in, 2 out]
                              }
                              frame "NEXT" {
                                n295 = invoke class="TrioPC" method="Execute"(reference=w567, error in=w566, "Command"="OP(55,ON)") -> (reference out=w565:refnum<k7>, error out=w564:errorcluster)  [unwired: 1 in, 2 out]
                              }
                            }
                          }
                          frame 1 {
                            n296 = invoke class="TrioPC" method="Execute"(reference=w571, error in=w570, "Command"="OP(53,ON)") -> (reference out=w568:refnum<k7>, error out=w569:errorcluster)  [unwired: 1 in, 2 out]
                          }
                          frame 2 {
                            n297 = invoke class="TrioPC" method="Execute"(reference=w577, error in=w576, "Command"="OP(52,ON)") -> (reference out=w575:refnum<k7>, error out=w574:errorcluster)  [unwired: 1 in, 2 out]
                          }
                          frame 3 {
                            n298 = invoke class="TrioPC" method="Execute"(reference=w581, error in=w582, "Command"="OP(50,ON)") -> (reference out=w580:refnum<k7>, error out=w579:errorcluster)  [unwired: 1 in, 2 out]
                          }
                          frame 4 {
                            n299 = invoke class="TrioPC" method="Execute"(reference=w587, error in=w586, "Command"="OP(51,ON)") -> (reference out=w585:refnum<k7>, error out=w584:errorcluster)  [unwired: 1 in, 2 out]
                          }
                          frame 5 {
                            n300 = invoke class="TrioPC" method="Execute"(reference=w592, error in=w591, "Command"="OP(54,ON)") -> (reference out=w590:refnum<k7>, error out=w589:errorcluster)  [unwired: 1 in, 2 out]
                          }
                          frame 6 {
                            n301 = invoke class="TrioPC" method="Execute"(reference=w597, error in=w596, "Command"="OP(55,ON)") -> (reference out=w595:refnum<k7>, error out=w594:errorcluster)  [unwired: 1 in, 2 out]
                          }
                        }
                      }
                    }
                    n302 = case shown="True" "Move" {
                      tunnel: [w673 w675] -> w470
                      tunnel: [w672 w674] -> w471
                      tunnel: w477 -> [w673 w678]
                      tunnel: w476 -> [w672 w677]
                      frame False {
                      }
                      frame True {
                        n303 = Build Array("Axis 0 Distance", "Axis 1 Distance", "Axis 2 Distance") -> (w676:dbl[])
                        n304 = case shown="\"Absolute\"" "Menu Ring" {
                          tunnel: w678 -> [w689 w695]
                          tunnel: w677 -> [w688 w694]
                          tunnel: w676 -> [w686 w691]
                          tunnel: [w684 w692] -> w675
                          tunnel: [w683 w693] -> w674
                          frame "Relative", Default {
                            n305 = invoke class="TrioPC" method="MoveRel"(reference=w689, error in=w688, "Axes"=i16 3, "Distance"=w686, "Axis"=0) -> (reference out=w684:refnum<k7>, error out=w683:errorcluster)  [unwired: 1 in, 4 out]
                          }
                          frame "Absolute" {
                            n306 = invoke class="TrioPC" method="MoveAbs"(reference=w695, error in=w694, "Axes"=i16 3, "Position"=w691, "Axis"=i16 0 ("Axes")) -> (reference out=w692:refnum<k7>, error out=w693:errorcluster)  [unwired: 1 in, 4 out]
                          }
                        }
                      }
                    }
                    n307 = Merge Errors(w471, w466) -> (w473:errorcluster)
                  }
                  frame "MEASUREMENT" {
                    n308 = case shown="0, Default" w701 {
                      tunnel: w708 -> [w718 _]
                      tunnel: w707 -> [_ w720]
                      tunnel: [w717 w719] -> w699
                      frame 0, Default {
                        n309 = Absolute Value(x=w718) -> (abs(x)=w717:dbl)
                      }
                      frame 1 {
                        n310 = Absolute Value(x=w720) -> (abs(x)=w719:dbl)
                      }
                    }
                    n311 = local read "Travel Dist"() -> (w712:dbl)
                    n312 = Equal To 0?(x=w699) -> (x = 0?=w700:bool)
                    n313 = case shown="2" w715 {
                      tunnel: w710 -> [w726 w778 w798 w857 w862]
                      tunnel: w709 -> [w725 w779 w799 w856 w861]
                      tunnel: w701 -> [_ w777 w800 w847 _]
                      tunnel: [w728 w776 w796 w854 w859] -> w706
                      tunnel: [w727 w775 w797 w855 w860] -> w711
                      tunnel: [w733 w773 w804 4 ("Measurement\nAxis") w863] -> w716
                      tunnel: w714 -> [_ w772 w794 w845 w865]
                      tunnel: [w732 w772 w794 w845 w864] -> w713
                      tunnel: w700 -> [_ _ w805 _ w866]
                      tunnel: w699 -> [_ _ w803 _ _]
                      tunnel: "Ramp Distance\n(mm)" -> [w724 _ w802 _ _]
                      tunnel: w712 -> [_ w771 w801 w844 _]
                      tunnel: "Travel Acc\n(mm/s2)" -> [w731 _ _ _ _]
                      tunnel: "Travel Speed\n(mm/s)" -> [w730 _ _ _ w858]
                      tunnel: "Evaluation Length\n(mm)" -> [w729 _ _ _ _]
                      tunnel: "Num Tracks" -> [w722 _ w795 _ _]
                      tunnel: "Sensor" -> [_ _ w791 _ _]
                      frame 0, Default {
                        # "Not Measuring"
                        n314 = case shown="True" "Set Parameters" {
                          tunnel: [w740 w755] -> w727
                          tunnel: [w739 w754] -> w728
                          tunnel: w726 -> [w740 w753]
                          tunnel: w725 -> [w739 w752]
                          tunnel: w731 -> [_ w748]
                          tunnel: w730 -> [_ w747]
                          tunnel: w729 -> [_ w741]
                          tunnel: w724 -> [_ w746]
                          frame False {
                          }
                          frame True {
                            n315 = Absolute Value(x=w746) -> (abs(x)=w750:dbl)
                            n316 = Absolute Value(x=w741) -> (abs(x)=w745:dbl)
                            n317 = for {
                              N: 2 -> [_]
                              tunnel: w747 -> [w763]
                              tunnel: w748 -> [w762]
                              shift-right: [w757] -> w754
                              shift-left: w752 -> [w759]
                              shift-right: [w758] -> w755
                              shift-left: w753 -> [w760]
                              i -> [w761]
                              n318 = invoke class="TrioPC" method="SetAxisVariable"(reference=w760, error in=w759, "Variable"="SPEED", "Axis"=w761, "Value"=w763) -> (reference out=w769:refnum<k7>, error out=w768:errorcluster)  [unwired: 1 in, 4 out]
                              n319 = invoke class="TrioPC" method="SetAxisVariable"(reference=w769, error in=w768, "Variable"="ACCEL", "Axis"=w761, "Value"=w762) -> (reference out=w767:refnum<k7>, error out=w766:errorcluster)  [unwired: 1 in, 4 out]
                              n320 = invoke class="TrioPC" method="SetAxisVariable"(reference=w767, error in=w766, "Variable"="DECEL", "Axis"=w761, "Value"=w762) -> (reference out=w758:refnum<k7>, error out=w757:errorcluster)  [unwired: 1 in, 4 out]
                            }
                            n321 = Multiply(x=w750, y=2.0) -> (x*y=w744:dbl)
                            n322 = Add(x=w744, y=w745) -> (x+y=w743:dbl)
                            n323 = Sign(1:w741) -> (0:w742:dbl)
                            n324 = Multiply(x=w743, y=w742) -> (x*y=→"Travel Dist":dbl)
                          }
                        }
                        n325 = case shown="True" "Start Measurement" {
                          tunnel: [0 ("Axes") 1 ("Axes")] -> w733
                          tunnel: [0 ("f") w738] -> w732
                          tunnel: w722 -> [_ w738]
                          frame False {
                          }
                          frame True {
                            n326 = local write "Setup Tab"(enum32{"SETUP", "MONITORING", "ERRORS"}."MONITORING" ("Setup Tab")) -> ()
                          }
                        }
                      }
                      frame 1 {
                        # "Start Measurement Sequence"
                        n327 = Not Equal To 0?(x=w772) -> (x != 0?=w774:bool)
                        n328 = case shown="True" w774 {
                          tunnel: w779 -> [w780 w790]
                          tunnel: w778 -> [w781 w789]
                          tunnel: w777 -> [_ w788]
                          tunnel: [w780 w787] -> w776
                          tunnel: [w781 w786] -> w775
                          tunnel: [0 ("Axes") 2 ("Axes")] -> w773
                          tunnel: w771 -> [_ w783]
                          frame False {
                            # "Return to Idle State"
                            # "No Tracks to measure"
                          }
                          frame True {
                            n329 = invoke class="TrioPC" method="MoveRel"(reference=w789, error in=w790, "Axes"=i16 1, "Distance"=w783, "Axis"=w788) -> (reference out=w786:refnum<k7>, error out=w787:errorcluster)  [unwired: 1 in, 4 out]
                          }
                        }
                      }
                      frame 2 {
                        # "Wait for Motion to Stop"
                        n330 = Subtract(x=w795, y=w794) -> (x-y=w793:i32)
                        n331 = Increment(x=w793) -> (x+1=w792:i32)
                        n332 = case shown="True" w805 {
                          tunnel: [2 ("Measurement\nAxis") 3 ("Measurement\nAxis")] -> w804
                          tunnel: w803 -> [w816 _]
                          tunnel: w802 -> [w815 _]
                          tunnel: w801 -> [w811 _]
                          tunnel: w800 -> [_ _]
                          tunnel: w799 -> [w809 w833]
                          tunnel: w798 -> [w808 w835]
                          tunnel: [w808 w832] -> w797
                          tunnel: [w809 w831] -> w796
                          tunnel: w792 -> [w807 _]
                          tunnel: w791 -> [w806 _]
                          frame False {
                            # "Axis Moving"
                            n333 = Absolute Value(x=w811) -> (abs(x)=w810:dbl)
                            n334 = Subtract(x=w810, y=w815) -> (x-y=w817:dbl)
                            n335 = Less Or Equal?(x=w816, y=w817) -> (x <= y?=w814:bool)
                            n336 = Greater Or Equal?(x=w816, y=w815) -> (x >= y?=w813:bool)
                            n337 = And(x=w814, y=w813) -> (x .and. y?=w812:bool)
                            n338 = case shown="False" w812 {
                              tunnel: w807 -> [_ w826]
                              tunnel: w806 -> [w819 w822]
                              frame False {
                                # "Axis Ramping Up / Down"
                                n339 = case shown="0, Default" w819 {
                                frame 0, Default {
                                n340 = local write "Chromatic Data \nLogging"(FALSE ("Log Chromatic Data")) -> ()
                                }
                                frame 1 {
                                n341 = local write "Laser Data\nLogging"(FALSE ("Log Chromatic Data")) -> ()
                                }
                                }
                              }
                              frame True {
                                # "Take Measurements"
                                n342 = Format Into String(format string="%02d", initial string="_", w826) -> (resulting string=→"Suffix":string)  [unwired: 1 in, 1 out]
                                n343 = case shown="0, Default" w822 {
                                frame 0, Default {
                                n344 = local write "Chromatic Data \nLogging"(TRUE ("Log Chromatic Data")) -> ()
                                }
                                frame 1 {
                                n345 = local write "Laser Data\nLogging"(TRUE ("Log Chromatic Data")) -> ()
                                }
                                }
                              }
                            }
                          }
                          frame True {
                            # "For instances when no ramp distance specified"
                            # "Increase speed for return motion"
                            # "Measurement Finished"
                            n346 = for {
                              N: 2 -> [_]
                              tunnel: w835 -> [w842]
                              tunnel: [w838] -> w832
                              shift-right: [w837] -> w831
                              shift-left: w833 -> [w843]
                              i -> [w841]
                              n347 = invoke class="TrioPC" method="SetAxisVariable"(reference=w842, error in=w843, "Variable"="SPEED", "Axis"=w841, "Value"=5.0) -> (reference out=w838:refnum<k7>, error out=w837:errorcluster)  [unwired: 1 in, 4 out]
                            }
                            n348 = local write "Chromatic Data \nLogging"(FALSE ("Chromatic Data \nLogging")) -> ()
                            n349 = local write "Laser Data\nLogging"(FALSE ("Laser Data\nLogging")) -> ()
                          }
                        }
                      }
                      frame 3 {
                        # "Return to start position / start of next track"
                        n350 = Build Array("Track Offset\n(mm)") -> (w851:dbl[])
                        n351 = Negate(x=w844) -> (-x=w852:dbl)
                        n352 = Insert Into Array(array=w851, index=w847, new element=w852) -> (w850:dbl[])
                        n353 = invoke class="TrioPC" method="MoveRel"(reference=w857, error in=w856, "Axes"=i16 2, "Distance"=w850, "Axis"=i16 0 ("Axes")) -> (reference out=w855:refnum<k7>, error out=w854:errorcluster)  [unwired: 1 in, 4 out]
                      }
                      frame 4 {
                        # "Wait until returned and axes stopped"
                        n354 = case shown="True" w866 {
                          tunnel: w865 -> [w870 w879]
                          tunnel: [w870 w878] -> w864
                          tunnel: [4 ("Measurement\nAxis") 1 ("Measurement\nAxis")] -> w863
                          tunnel: w862 -> [w868 w875]
                          tunnel: w861 -> [w867 w874]
                          tunnel: [w868 w873] -> w860
                          tunnel: [w867 w872] -> w859
                          tunnel: w858 -> [_ w871]
                          frame False {
                            # "Still Moving"
                          }
                          frame True {
                            # "Start next measurement"
                            # "Finished Movement"
                            n355 = for {
                              N: 2 -> [_]
                              tunnel: w875 -> [w885]
                              tunnel: [w882] -> w873
                              shift-right: [w881] -> w872
                              shift-left: w874 -> [w886]
                              tunnel: w871 -> [w880]
                              i -> [w884]
                              n356 = invoke class="TrioPC" method="SetAxisVariable"(reference=w885, error in=w886, "Variable"="SPEED", "Axis"=w884, "Value"=w880) -> (reference out=w882:refnum<k7>, error out=w881:errorcluster)  [unwired: 1 in, 4 out]
                            }
                            n357 = Decrement(x=w879) -> (x-1=w878:i32)
                          }
                        }
                      }
                    }
                  }
                }
                n358 = invoke class="TrioPC" method="GetAxisVariable"(reference=w336, error in=w373, "Variable"="AXISSTATUS", "Axis"=i16 0) -> (reference out=w372:refnum<k7>, error out=w365:errorcluster, "Value"=w367:dbl)  [unwired: 2 in, 3 out]
                n359 = invoke class="TrioPC" method="GetAxisVariable"(reference=w336, "Variable"="AXISSTATUS", "Axis"=i16 1) -> ("Value"=w366:dbl)  [unwired: 3 in, 5 out]
                n360 = invoke class="TrioPC" method="GetAxisVariable"(reference=w336, "Variable"="AXISSTATUS", "Axis"=i16 2) -> ("Value"=w364:dbl)  [unwired: 3 in, 5 out]
                n361 = invoke class="TrioPC" method="GetAxisVariable"(reference=w336, "Variable"="MPOS", "Axis"=i16 3) -> ("Value"=→"Encoder Value":dbl)  [unwired: 3 in, 5 out]
                n362 = call "Controller - Generate Axis Error.vi"("Error Code"=w367) -> ("Error Description"=w357:errorcluster)
                "X Axis Error" <- w357
                n363 = call "Controller - Generate Axis Error.vi"("Error Code"=w366) -> ("Error Description"=w356:errorcluster)
                "Y Axis Error" <- w356
                n364 = call "Controller - Generate Axis Error.vi"("Error Code"=w364) -> ("Error Description"=w361:errorcluster)
                "Z Axis Error" <- w361
                n365 = Unbundle By Name(w357) -> ("status"=→"X Error":bool)
                n366 = Unbundle By Name(w356) -> ("status"=→"Y Error":bool)
                n367 = Unbundle By Name(w361) -> ("status"=→"Z Error":bool)
              }
            }
          }
        }
        "Controller  Error" <- w231
        n368 = To Double Precision Float(number=w232) -> (double precision float=w235:dbl)
        n369 = Divide(x=w235, y=1000.0) -> (x/y=w239:dbl)
        n370 = To Long Integer(number=w239) -> (32bit integer=→"Total Time Elapsed (s)":i32)
      }
      n371 = call "Imaq Dispose"("Image"=w19) -> ()  [unwired: 5 in, 1 out]
      n372 = case shown="True" w27 {
        tunnel: w24 -> [_ w890]
        tunnel: w25 -> [w887 w888]
        tunnel: [w887 w889] -> w26
        frame False {
        }
        frame True {
          n373 = call <vilib>:"IMAQdx Close Camera.vi"("error in"=w888, "Session In"=w890) -> ("error out"=w889:errorcluster)  [unwired: 9 out]
        }
      }
      n374 = call <vilib>:"Simple Error Handler.vi"("error in (no error)"=w26) -> ()  [unwired: 4 in, 5 out]
    }
    frame #2 {
      n375 = call-poly <vilib>:"Close Input Device.vi"("device ID"=w1154) -> ()  [unwired: 9 in, 1 out]
      n376 = invoke class="TrioPC" method="Execute"(reference=w1152, error in=w1153, "Command"="RAPIDSTOP(2)") -> (reference out=w1148:refnum<k7>, error out=w1149:errorcluster)  [unwired: 1 in, 2 out]
      n377 = invoke class="TrioPC" method="SetVariable"(reference=w1148, error in=w1149, "Variable"="WDOG", "Value"=0.0) -> (reference out=w1147:refnum<k7>, error out=w1146:errorcluster)  [unwired: 1 in, 3 out]
      n378 = invoke class="TrioPC" method="Close"(reference=w1147, error in=w1146) -> (reference out=w1155:refnum<k7>, error out=w1156:errorcluster)  [unwired: 2 in, 2 out]
      n379 = Close Reference(reference=w1155, error in (no error)=w1156) -> (error out=w1151:errorcluster)
      n380 = call <vilib>:"Simple Error Handler.vi"("error in (no error)"=w1151) -> ()  [unwired: 4 in, 5 out]
    }
  }
